vi "DblMonoPMDCurrentScanSM correction 2.vi"() -> ()   [LabVIEW 2009]
uses:
  <vilib>/DAQmx/create/channels.llb/DAQmx Create Channel (AI-Voltage-Basic).vi
  <vilib>/DAQmx/create/channels.llb/DAQmx Create Channel (AO-Voltage-Basic).vi
  <vilib>/DAQmx/write.llb/DAQmx Write (Analog DBL 1Chan 1Samp).vi
  <vilib>/DAQmx/read.llb/DAQmx Read (Analog 1D DBL 1Chan NSamp).vi
  <vilib>/DAQmx/configure/timing.llb/DAQmx Timing (Sample Clock).vi
  <vilib>/DAQmx/read.llb/DAQmx Read (Analog 1D DBL NChan 1Samp).vi
  <vilib>/DAQmx/write.llb/DAQmx Write (Analog 1D DBL 1Chan NSamp).vi
  <vilib>/Utility/file.llb/Write To Spreadsheet File (DBL).vi
  <vilib>/Analysis/NI_AALBase.lvlib
panel:
  in  "Scan mirrors out 2":tag
  out "initial y 2":dbl
  out "Final Y 2":dbl
  out "Final Y":dbl
  out "initial y":dbl
  in  "Volts/pixel":dbl
  out "Xin":dbl
  out "Yin":dbl
  in  "Correction":dbl[][](array[numeric])
  in  "Scan mirrors out":tag
  in  "Scan Mirrors in":tag
  in  "Voltage B":dbl min=-10.0 max=10.0 step=0.1 format="%0.2f"
  in  "Voltage A":dbl min=-10.0 max=10.0 step=0.1 format="%0.2f"
  in  "Output B":tag="Dev1/ao3"
  in  "Output A":tag="Dev1/ao2"
  in  "Input Channel":tag="Dev1/ai6"
  in  "Current":bool
  in  "Power":bool=TRUE
  out "ScanGraph":cluster{dbl[], dbl[]}(graph)
  in  "Sensitivity":dbl=1e-09 caption="(A/V)" format="%#_6p"
  out "Readout":dbl=-2.45576047e-07 format="%^#_9e"
  in  "Scan Save Path":path
  in  "On":bool=TRUE
  out "Waveform Chart":dbl(graph)=-2.45576047e-07
  in  "Save":bool=TRUE
  in  "Exit":bool
  in  "STOP":bool
  in  "Step Time (sec)":dbl=1.0 min=0.001 max=300.0 step=0.001 format="%.3f"
  in  "Step Size (nm)":dbl=1.0 min=0.1 max=100.0 step=0.1 format="%.1f"
  in  "End":dbl=800.0 min=0.0 max=2000.0 step=0.1 format="%.1f"
  in  "Start":dbl=400.0 min=0.0 max=2000.0 step=0.1 format="%.1f"
  in  "Scan":bool
  in  "Up":bool=TRUE caption="Down"
  in  "Increment (nm)":dbl=10.0 min=0.1 max=2000.0 step=0.1 format="%.1f"
  in  "PMD Settings":T1={"Beam Diameter (mm)"=4.0, "BWIn"=0, "Averaging Rate"=300, "Auto Range"=TRUE} {"Averaging Rate" min=33 max=5000 step=1; "BWIn" items=["HIGH", "LOW"]; "Beam Diameter (mm)" min=1.0 max=9.0 step=0.5}
  in  "Step":bool
  out "Busy":bool=TRUE
  in  "Send Command":bool
  in  "Command":u16(ring)=1 items=["nm", "goto", "nm/min", "VIS grating", "IR grating"]
  in  "Wavelength (nm)":dbl=500.0 min=0.0 max=2000.0 step=0.1 format="%.1f"
  in  "Scan Speed (nm/min)":dbl=100.0 min=1.0 max=500.0 step=0.1 format="%.1f"
  out "Done?":string="   ..."
  in  "Send Question":bool
  in  "Ask?":u16(ring) items=["?nm", "?nm/min", "?grating", "?turret", "?gratings"]
  in  "Zero?":bool
  out "PM Error log":string="-222,\"Data out of range\"\n-222,\"Data out of range\"\n-222,\"Data out of range\"\n-222,\"Data out of range\"\n-222,\"Data out of range\"\n-222,\"Data out of range\"\n-222,\"Data out of range\"\n-222,\"Data out of range\"\n-222,\"Data out of range\"\n-222,\"Data out of range\"\n-222,\"Data out of range\"\n-222,\"Data out of range\"\n-222,\"Data out of range\"\n-222,\"Data out of range\"\n-222,\"Data out of range\"\n-222,\"Data out of range\"\n-222,\"Data out of range\"\n-222,\"Data out of range\"\n-222,\"Data out of range\"\n-222,\"Data out of range\"\n-222,\"Data out of range\"\n-222,\"Data out of range\"\n-222,\"Data out of range\"\n-222,\"Data out of range\"\n-222,\"Data out of range\"\n-222,\"Data out of range\"\n-222,\"Data out of range\"\n-222,\"Data out of range\"\n-222,\"Data out of range\"\n-222,\"Data out of range\"\n-222,\"Data out of range\"\n-222,\"Data out of range\"\n-222,\"Data out of range\"\n-222,\"Data out of range\"\n-222,\"Data out of range\"\n-222,\"Data out of range\"\n-222,\"Data out of range\"\n-222,\"Data out of range\"\n-222,\"Data out of range\"\n-222,\"Data out of range\"\n-222,\"Data out of range\"\n-222,\"Data out of range\"\n-222,\"Data out of range\"\n-222,\"Data out of range\"\n-222,\"Data out of range\"\n-222,\"Data out of range\"\n-222,\"Data out of range\"\n-222,\"Data out of range\"\n-222,\"Data out of range\"\n-222,\"Data out of range\"\n-222,\"Data out of range\"\n-222,\"Data out of range\"\n-222,\"Data out of range\"\n-222,\"Data out of range\"\n-222,\"Data out of range\"\n-222,\"Data out of range\"\n-222,\"Data out of range\"\n-222,\"Data out of range\"\n-222,\"Data out of range\"\n-222,\"Data out of range\"\n-222,\"Data out of range\"\n-222,\"Data out of range\"\n-222,\"Data out of range\"\n-222,\"Data out of range\"\n-222,\"Data out of range\"\n-222,\"Data out of range\"\n-222,\"Data out of range\"\n-222,\"Data out of range\"\n-222,\"Data out of range\"\n-222,\"Data out of range\"\n-222,\"Data out of range\"\n-222,\"Data out of range\"\n-222,\"Data out of range\"\n-222,\"Data out of range\"\n-222,\"Data out of range\"\n-222,\"Data out of range\"\n-222,\"Data out of range\"\n-222,\"Data out of range\"\n-222,\"Data out of range\"\n-222,\"Data out of range\"\n-222,\"Data out of range\"\n-222,\"Data out of range\"\n-222,\"Data out of range\"\n-222,\"Data out of range\"\n-222,\"Data out of range\"\n-222,\"Data out of range\"\n-222,\"Data out of range\"\n-222,\"Data out of range\"\n-222,\"Data out of range\"\n-222,\"Data out of range\"\n-222,\"Data out of range\"\n-222,\"Data out of range\"\n-222,\"Data out of range\"\n-222,\"Data out of range\"\n-222,\"Data out of range\"\n-222,\"Data out of range\"\n-222,\"Data out of range\"\n-222,\"Data out of range\"\n-222,\"Data out of range\"\n-222,\"Data out of range\"\n-222,\"Data out of range\"\n-222,\"Data out of range\"\n-222,\"Data out of range\"\n-222,\"Data out of range\"\n-222,\"Data out of range\"\n-222,\"Data out of range\"\n-222,\"Data out of range\"\n-222,\"Data out of range\"\n-222,\"Data out of range\"\n-222,\"Data out of range\"\n-222,\"Data out of range\"\n-222,\"Data out of range\"\n-222,\"Data out of range\"\n-222,\"Data out of range\"\n-222,\"Data out of range\"\n-222,\"Data out of range\"\n-222,\"Data out of range\"\n-222,\"Data out of range\"\n-222,\"Data out of range\"\n-222,\"Data out of range\"\n-222,\"Data out of range\"\n-222,\"Data out of range\"\n-222,\"Data out of range\"\n-222,\"Data out of range\"\n-222,\"Data out of range\"\n-222,\"Data out of range\"\n-222,\"Data out of range\"\n-222,\"Data out of range\"\n-222,\"Data out of range\"\n-222,\"Data out of range\"\n-222,\"Data out of range\"\n-222,\"Data out of range\"\n-222,\"Data out of range\"\n-222,\"Data out of range\"\n-222,\"Data out of range\"\n-222,\"Data out of range\"\n-222,\"Data out of range\"\n-222,\"Data out of range\"\n-222,\"Data out of range\"\n-222,\"Data out of range\"\n-222,\"Data out of range\"\n-222,\"Data out of range\"\n-222,\"Data out of range\"\n-222,\"Data out of range\"\n-222,\"Data out of range\"\n-222,\"Data out of range\"\n-222,\"Data out of range\"\n-222,\"Data out of range\"\n-222,\"Data out of range\"\n-222,\"Data out of range\"\n-222,\"Data out of range\"\n-222,\"Data out of range\"\n-222,\"Data out of range\"\n-222,\"Data out of range\"\n-222,\"Data out of range\"\n-222,\"Data out of range\"\n-222,\"Data out of range\"\n-222,\"Data out of range\"\n-222,\"Data out of range\"\n-222,\"Data out of range\"\n-222,\"Data out of range\"\n-222,\"Data out of range\"\n-222,\"Data out of range\"\n-222,\"Data out of range\"\n-222,\"Data out of range\"\n-222,\"Data out of range\"\n-222,\"Data out of range\"\n-222,\"Data out of range\"\n-222,\"Data out of range\"\n-222,\"Data out of range\"\n-222,\"Data out of range\"\n-222,\"Data out of range\"\n-222,\"Data out of range\"\n-222,\"Data out of range\"\n-222,\"Data out of range\"\n-222,\"Data out of range\"\n-222,\"Data out of range\"\n-222,\"Data out of range\"\n-222,\"Data out of range\"\n-222,\"Data out of range\"\n-222,\"Data out of range\"\n-222,\"Data out of range\"\n-222,\"Data out of range\"\n-222,\"Data out of range\"\n-222,\"Data out of range\"\n-222,\"Data out of range\"\n-222,\"Data out of range\"\n-222,\"Data out of range\"\n-222,\"Data out of range\"\n-222,\"Data out of range\"\n-222,\"Data out of range\"\n-222,\"Data out of range\"\n-222,\"Data out of range\"\n-222,\"Data out of range\"\n-222,\"Data out of range\"\n-222,\"Data out of range\"\n-222,\"Data out of range\"\n-222,\"Data out of range\"\n-222,\"Data out of range\"\n-222,\"Data out of range\"\n-222,\"Data out of range\"\n-222,\"Data out of range\"\n-222,\"Data out of range\"\n-222,\"Data out of range\"\n-222,\"Data out of range\"\n-222,\"Data out of range\"\n-222,\"Data out of range\"\n-222,\"Data out of range\"\n-222,\"Data out of range\"\n-222,\"Data out of range\"\n-222,\"Data out of range\"\n-222,\"Data out of range\"\n-222,\"Data out of range\"\n-222,\"Data out of range\"\n-222,\"Data out of range\"\n-222,\"Data out of range\"\n-222,\"Data out of range\"\n-222,\"Data out of range\"\n-222,\"Data out of range\"\n-222,\"Data out of range\"\n-222,\"Data out of range\"\n-222,\"Data out of range\"\n-222,\"Data out of range\"\n-222,\"Data out of range\"\n-222,\"Data out of range\"\n-222,\"Data out of range\"\n-222,\"Data out of range\"\n-222,\"Data out of range\"\n-222,\"Data out of range\"\n-222,\"Data out of range\"\n-222,\"Data out of range\"\n-222,\"Data out of range\"\n-222,\"Data out of range\"\n-222,\"Data out of range\"\n-222,\"Data out of range\"\n-222,\"Data out of range\"\n-222,\"Data out of range\"\n-222,\"Data out of range\"\n-222,\"Data out of range\"\n-222,\"Data out of range\"\n-222,\"Data out of range\"\n-222,\"Data out of range\"\n-222,\"Data out of range\"\n-222,\"Data out of range\"\n-222,\"Data out of range\"\n-222,\"Data out of range\"\n-222,\"Data out of range\"\n-222,\"Data out of range\"\n-222,\"Data out of range\"\n-222,\"Data out of range\"\n-222,\"Data out of range\"\n-222,\"Data out of range\"\n-222,\"Data out of range\"\n-222,\"Data out of range\"\n-222,\"Data out of range\"\n-222,\"Data out of range\"\n-222,\"Data out of range\"\n-222,\"Data out of range\"\n-222,\"Data out of range\"\n-222,\"Data out of range\"\n-222,\"Data out of range\"\n-222,\"Data out of range\"\n-222,\"Data out of range\"\n-222,\"Data out of range\"\n-222,\"Data out of range\"\n-222,\"Data out of range\"\n-222,\"Data out of range\"\n-222,\"Data out of range\"\n-222,\"Data out of range\"\n-222,\"Data out of range\"\n-222,\"Data out of range\"\n-222,\"Data out of range\"\n-222,\"Data out of range\"\n-222,\"Data out of range\"\n-222,\"Data out of range\"\n-222,\"Data out of range\"\n-222,\"Data out of range\"\n-222,\"Data out of range\"\n-222,\"Data out of range\"\n-222,\"Data out of range\"\n-222,\"Data out of range\"\n-222,\"Data out of range\"\n-222,\"Data out of range\"\n-222,\"Data out of range\"\n-222,\"Data out of range\"\n-222,\"Data out of range\"\n-222,\"Data out of range\"\n-222,\"Data out of range\"\n-222,\"Data out of range\"\n-222,\"Data out of range\"\n-222,\"Data out of range\"\n-222,\"Data out of range\"\n-222,\"Data out of range\"\n-222,\"Data out of range\"\n-222,\"Data out of range\"\n-222,\"Data out of range\"\n-222,\"Data out of range\"\n-222,\"Data out of range\"\n-222,\"Data out of range\"\n-222,\"Data out of range\"\n-222,\"Data out of range\"\n-222,\"Data out of range\"\n-222,\"Data out of range\"\n-222,\"Data out of range\"\n-222,\"Data out of range\"\n-222,\"Data out of range\"\n-222,\"Data out of range\"\n-222,\"Data out of range\"\n-222,\"Data out of range\"\n-222,\"Data out of range\"\n-222,\"Data out of range\"\n-222,\"Data out of range\"\n-222,\"Data out of range\"\n-222,\"Data out of range\"\n-222,\"Data out of range\"\n-222,\"Data out of range\"\n-222,\"Data out of range\"\n-222,\"Data out of range\"\n-222,\"Data out of range\"\n-222,\"Data out of range\"\n-222,\"Data out of range\"\n-222,\"Data out of range\"\n-222,\"Data out of range\"\n-222,\"Data out of range\"\n-222,\"Data out of range\"\n-222,\"Data out of range\"\n-222,\"Data out of range\"\n-222,\"Data out of range\"\n-222,\"Data out of range\"\n-222,\"Data out of range\"\n-222,\"Data out of range\"\n-222,\"Data out of range\"\n-222,\"Data out of range\"\n-222,\"Data out of range\"\n-222,\"Data out of range\"\n-222,\"Data out of range\"\n-222,\"Data out of range\"\n-222,\"Data out of range\"\n-222,\"Data out of range\"\n-222,\"Data out of range\"\n-222,\"Data out of range\"\n-222,\"Data out of range\"\n-222,\"Data out of range\"\n-222,\"Data out of range\"\n-222,\"Data out of range\"\n-222,\"Data out of range\"\n-222,\"Data out of range\"\n-222,\"Data out of range\"\n-222,\"Data out of range\"\n-222,\"Data out of range\"\n-222,\"Data out of range\"\n-222,\"Data out of range\"\n-222,\"Data out of range\"\n-222,\"Data out of range\"\n-222,\"Data out of range\"\n-222,\"Data out of range\"\n-222,\"Data out of range\"\n-222,\"Data out of range\"\n-222,\"Data out of range\"\n-222,\"Data out of range\"\n-222,\"Data out of range\"\n-222,\"Data out of range\"\n-222,\"Data out of range\"\n-222,\"Data out of range\"\n-222,\"Data out of range\"\n-222,\"Data out of range\"\n-222,\"Data out of range\"\n-222,\"Data out of range\"\n-222,\"Data out of range\"\n-222,\"Data out of range\"\n-222,\"Data out of range\"\n-222,\"Data out of range\"\n-222,\"Data out of range\"\n-222,\"Data out of range\"\n-222,\"Data out of range\"\n-222,\"Data out of range\"\n-222,\"Data out of range\"\n-222,\"Data out of range\"\n-222,\"Data out of range\"\n-222,\"Data out of range\"\n-222,\"Data out of range\"\n-222,\"Data out of range\"\n-222,\"Data out of range\"\n-222,\"Data out of range\"\n-222,\"Data out of range\"\n-222,\"Data out of range\"\n-222,\"Data out of range\"\n-222,\"Data out of range\"\n-222,\"Data out of range\"\n-222,\"Data out of range\"\n-222,\"Data out of range\"\n-222,\"Data out of range\"\n-222,\"Data out of range\"\n-222,\"Data out of range\"\n-222,\"Data out of range\"\n-222,\"Data out of range\"\n-222,\"Data out of range\"\n-222,\"Data out of range\"\n-222,\"Data out of range\"\n-222,\"Data out of range\"\n-222,\"Data out of range\"\n-222,\"Data out of range\"\n-222,\"Data out of range\"\n-222,\"Data out of range\"\n-222,\"Data out of range\"\n-222,\"Data out of range\"\n-222,\"Data out of range\"\n-222,\"Data out of range\"\n-222,\"Data out of range\"\n-222,\"Data out of range\"\n-222,\"Data out of range\"\n-222,\"Data out of range\"\n-222,\"Data out of range\"\n-222,\"Data out of range\"\n-222,\"Data out of range\"\n-222,\"Data out of range\"\n-222,\"Data out of range\"\n-222,\"Data out of range\"\n-222,\"Data out of range\"\n-222,\"Data out of range\"\n-222,\"Data out of range\"\n-222,\"Data out of range\"\n-222,\"Data out of range\"\n-222,\"Data out of range\"\n-222,\"Data out of range\"\n-222,\"Data out of range\"\n-222,\"Data out of range\"\n-222,\"Data out of range\"\n-222,\"Data out of range\"\n-222,\"Data out of range\"\n-222,\"Data out of range\"\n-222,\"Data out of range\"\n-222,\"Data out of range\"\n-222,\"Data out of range\"\n-222,\"Data out of range\"\n-222,\"Data out of range\"\n-222,\"Data out of range\"\n-222,\"Data out of range\"\n-222,\"Data out of range\"\n-222,\"Data out of range\"\n-222,\"Data out of range\"\n-222,\"Data out of range\"\n-222,\"Data out of range\"\n-222,\"Data out of range\"\n-222,\"Data out of range\"\n-222,\"Data out of range\"\n-222,\"Data out of range\"\n-222,\"Data out of range\"\n-222,\"Data out of range\"\n-222,\"Data out of range\"\n-222,\"Data out of range\"\n-222,\"Data out of range\"\n-222,\"Data out of range\"\n-222,\"Data out of range\"\n-222,\"Data out of range\"\n-222,\"Data out of range\"\n-222,\"Data out of range\"\n-222,\"Data out of range\"\n-222,\"Data out of range\"\n-222,\"Data out of range\"\n-222,\"Data out of range\"\n-222,\"Data out of range\"\n-222,\"Data out of range\"\n-222,\"Data out of range\"\n-222,\"Data out of range\"\n-222,\"Data out of range\"\n-222,\"Data out of range\"\n-222,\"Data out of range\"\n-222,\"Data out of range\"\n-222,\"Data out of range\"\n-222,\"Data out of range\"\n-222,\"Data out of range\"\n-222,\"Data out of range\"\n-222,\"Data out of range\"\n-222,\"Data out of range\"\n-222,\"Data out of range\"\n-222,\"Data out of range\"\n-222,\"Data out of range\"\n-222,\"Data out of range\"\n-222,\"Data out of range\"\n-222,\"Data out of range\"\n-222,\"Data out of range\"\n-222,\"Data out of range\"\n-222,\"Data out of range\"\n-222,\"Data out of range\"\n-222,\"Data out of range\"\n-222,\"Data out of range\"\n-222,\"Data out of range\"\n-222,\"Data out of range\"\n-222,\"Data out of range\"\n-222,\"Data out of range\"\n-222,\"Data out of range\"\n-222,\"Data out of range\"\n-222,\"Data out of range\"\n-222,\"Data out of range\"\n-222,\"Data out of range\"\n-222,\"Data out of range\"\n-222,\"Data out of range\"\n-222,\"Data out of range\"\n-222,\"Data out of range\"\n-222,\"Data out of range\"\n-222,\"Data out of range\"\n-222,\"Data out of range\"\n-222,\"Data out of range\"\n-222,\"Data out of range\"\n-222,\"Data out of range\"\n-222,\"Data out of range\"\n-222,\"Data out of range\"\n-222,\"Data out of range\"\n-222,\"Data out of range\"\n-222,\"Data out of range\"\n-222,\"Data out of range\"\n-222,\"Data out of range\"\n-222,\"Data out of range\"\n-222,\"Data out of range\"\n-222,\"Data out of range\"\n-222,\"Data out of range\"\n-222,\"Data out of range\"\n-222,\"Data out of range\"\n-222,\"Data out of range\"\n-222,\"Data out of range\"\n-222,\"Data out of range\"\n-222,\"Data out of range\"\n-222,\"Data out of range\"\n-222,\"Data out of range\"\n-222,\"Data out of range\"\n-222,\"Data out of range\"\n-222,\"Data out of range\"\n-222,\"Data out of range\"\n-222,\"Data out of range\"\n-222,\"Data out of range\"\n-222,\"Data out of range\"\n-222,\"Data out of range\"\n-222,\"Data out of range\"\n-222,\"Data out of range\"\n-222,\"Data out of range\"\n-222,\"Data out of range\"\n-222,\"Data out of range\"\n-222,\"Data out of range\"\n-222,\"Data out of range\"\n-222,\"Data out of range\"\n-222,\"Data out of range\"\n-222,\"Data out of range\"\n-222,\"Data out of range\"\n-222,\"Data out of range\"\n-222,\"Data out of range\"\n-222,\"Data out of range\"\n-222,\"Data out of range\"\n-222,\"Data out of range\"\n-222,\"Data out of range\"\n-222,\"Data out of range\"\n-222,\"Data out of range\"\n-222,\"Data out of range\"\n-222,\"Data out of range\"\n-222,\"Data out of range\"\n-222,\"Data out of range\"\n-222,\"Data out of range\"\n-222,\"Data out of range\"\n-222,\"Data out of range\"\n-222,\"Data out of range\"\n-222,\"Data out of range\"\n-222,\"Data out of range\"\n-222,\"Data out of range\"\n-222,\"Data out of range\"\n-222,\"Data out of range\"\n-222,\"Data out of range\"\n-222,\"Data out of range\"\n-222,\"Data out of range\"\n-222,\"Data out of range\"\n-222,\"Data out of range\"\n-222,\"Data out of range\"\n-222,\"Data out of range\"\n-222,\"Data out of range\"\n-222,\"Data out of range\"\n-222,\"Data out of range\"\n-222,\"Data out of range\"\n-222,\"Data out of range\"\n-222,\"Data out of range\"\n-222,\"Data out of range\"\n-222,\"Data out of range\"\n-222,\"Data out of range\"\n-222,\"Data out of range\"\n-222,\"Data out of range\"\n-222,\"Data out of range\"\n-222,\"Data out of range\"\n-222,\"Data out of range\"\n-222,\"Data out of range\"\n-222,\"Data out of range\"\n-222,\"Data out of range\"\n-222,\"Data out of range\"\n-222,\"Data out of range\"\n-222,\"Data out of range\"\n-222,\"Data out of range\"\n-222,\"Data out of range\"\n-222,\"Data out of range\"\n-222,\"Data out of range\"\n-222,\"Data out of range\"\n-222,\"Data out of range\"\n-222,\"Data out of range\"\n-222,\"Data out of range\"\n-222,\"Data out of range\"\n-222,\"Data out of range\"\n-222,\"Data out of range\"\n-222,\"Data out of range\"\n-222,\"Data out of range\"\n-222,\"Data out of range\"\n-222,\"Data out of range\"\n-222,\"Data out of range\"\n-222,\"Data out of range\"\n-222,\"Data out of range\"\n-222,\"Data out of range\"\n-222,\"Data out of range\"\n-222,\"Data out of range\"\n-222,\"Data out of range\"\n-222,\"Data out of range\"\n-222,\"Data out of range\"\n-222,\"Data out of range\"\n-222,\"Data out of range\"\n-222,\"Data out of range\"\n-222,\"Data out of range\"\n-222,\"Data out of range\"\n-222,\"Data out of range\"\n-222,\"Data out of range\"\n-222,\"Data out of range\"\n-222,\"Data out of range\"\n-222,\"Data out of range\"\n-222,\"Data out of range\"\n-222,\"Data out of range\"\n-222,\"Data out of range\"\n-222,\"Data out of range\"\n-222,\"Data out of range\"\n-222,\"Data out of range\"\n-222,\"Data out of range\"\n-222,\"Data out of range\"\n-222,\"Data out of range\"\n-222,\"Data out of range\"\n-222,\"Data out of range\"\n-222,\"Data out of range\"\n-222,\"Data out of range\"\n-222,\"Data out of range\"\n-222,\"Data out of range\"\n-222,\"Data out of range\"\n-222,\"Data out of range\"\n-222,\"Data out of range\"\n-222,\"Data out of range\"\n-222,\"Data out of range\"\n-222,\"Data out of range\"\n-222,\"Data out of range\"\n-222,\"Data out of range\"\n-222,\"Data out of range\"\n-222,\"Data out of range\"\n-222,\"Data out of range\"\n-222,\"Data out of range\"\n-222,\"Data out of range\"\n-222,\"Data out of range\"\n-222,\"Data out of range\"\n-222,\"Data out of range\"\n-222,\"Data out of range\"\n-222,\"Data out of range\"\n-222,\"Data out of range\"\n-222,\"Data out of range\"\n-222,\"Data out of range\"\n-222,\"Data out of range\"\n-222,\"Data out of range\"\n-222,\"Data out of range\"\n-222,\"Data out of range\"\n-222,\"Data out of range\"\n-222,\"Data out of range\"\n-222,\"Data out of range\"\n-222,\"Data out of range\"\n-222,\"Data out of range\"\n-222,\"Data out of range\"\n-222,\"Data out of range\"\n-222,\"Data out of range\"\n-222,\"Data out of range\"\n-222,\"Data out of range\"\n-222,\"Data out of range\"\n-222,\"Data out of range\"\n-222,\"Data out of range\"\n-222,\"Data out of range\"\n-222,\"Data out of range\"\n-222,\"Data out of range\"\n-222,\"Data out of range\"\n-222,\"Data out of range\"\n-222,\"Data out of range\"\n-222,\"Data out of range\"\n-222,\"Data out of range\"\n-222,\"Data out of range\"\n-222,\"Data out of range\"\n-222,\"Data out of range\"\n-222,\"Data out of range\"\n-222,\"Data out of range\"\n-222,\"Data out of range\"\n-222,\"Data out of range\"\n-222,\"Data out of range\"\n-222,\"Data out of range\"\n-222,\"Data out of range\"\n-222,\"Data out of range\"\n-222,\"Data out of range\"\n-222,\"Data out of range\"\n-222,\"Data out of range\"\n-222,\"Data out of range\"\n-222,\"Data out of range\"\n-222,\"Data out of range\"\n-222,\"Data out of range\"\n-222,\"Data out of range\"\n-222,\"Data out of range\"\n-222,\"Data out of range\"\n-222,\"Data out of range\"\n-222,\"Data out of range\"\n-222,\"Data out of range\"\n-222,\"Data out of range\"\n-222,\"Data out of range\"\n-222,\"Data out of range\"\n-222,\"Data out of range\"\n-222,\"Data out of range\"\n-222,\"Data out of range\"\n-222,\"Data out of range\"\n-222,\"Data out of range\"\n-222,\"Data out of range\"\n-222,\"Data out of range\"\n-222,\"Data out of range\"\n-222,\"Data out of range\"\n-222,\"Data out of range\"\n-222,\"Data out of range\"\n-222,\"Data out of range\"\n-222,\"Data out of range\"\n-222,\"Data out of range\"\n-222,\"Data out of range\"\n-222,\"Data out of range\"\n-222,\"Data out of range\"\n-222,\"Data out of range\"\n-222,\"Data out of range\"\n-222,\"Data out of range\"\n-222,\"Data out of range\"\n-222,\"Data out of range\"\n-222,\"Data out of range\"\n-222,\"Data out of range\"\n-222,\"Data out of range\"\n-222,\"Data out of range\"\n-222,\"Data out of range\"\n-222,\"Data out of range\"\n-222,\"Data out of range\"\n-222,\"Data out of range\"\n-222,\"Data out of range\"\n-222,\"Data out of range\"\n-222,\"Data out of range\"\n-222,\"Data out of range\"\n-222,\"Data out of range\"\n-222,\"Data out of range\"\n-222,\"Data out of range\"\n-222,\"Data out of range\"\n-222,\"Data out of range\"\n-222,\"Data out of range\"\n-222,\"Data out of range\"\n-222,\"Data out of range\"\n-222,\"Data out of range\"\n-222,\"Data out of range\"\n-222,\"Data out of range\"\n-222,\"Data out of range\"\n-222,\"Data out of range\"\n-222,\"Data out of range\"\n-222,\"Data out of range\"\n-222,\"Data out of range\"\n-222,\"Data out of range\"\n-222,\"Data out of range\"\n-222,\"Data out of range\"\n-222,\"Data out of range\"\n-222,\"Data out of range\"\n-222,\"Data out of range\"\n-222,\"Data out of range\"\n-222,\"Data out of range\"\n-222,\"Data out of range\"\n-222,\"Data out of range\"\n-222,\"Data out of range\"\n-222,\"Data out of range\"\n-222,\"Data out of range\"\n-222,\"Data out of range\"\n-222,\"Data out of range\"\n-222,\"Data out of range\"\n-222,\"Data out of range\"\n-222,\"Data out of range\"\n-222,\"Data out of range\"\n-222,\"Data out of range\"\n-222,\"Data out of range\"\n-222,\"Data out of range\"\n-222,\"Data out of range\"\n-222,\"Data out of range\"\n-222,\"Data out of range\"\n-222,\"Data out of range\"\n-222,\"Data out of range\"\n-222,\"Data out of range\"\n-222,\"Data out of range\"\n-222,\"Data out of range\"\n-222,\"Data out of range\"\n-222,\"Data out of range\"\n-222,\"Data out of range\"\n-222,\"Data out of range\"\n-222,\"Data out of range\"\n-222,\"Data out of range\"\n-222,\"Data out of range\"\n-222,\"Data out of range\"\n-222,\"Data out of range\"\n-222,\"Data out of range\"\n-222,\"Data out of range\"\n-222,\"Data out of range\"\n-222,\"Data out of range\"\n-222,\"Data out of range\"\n-222,\"Data out of range\"\n-222,\"Data out of range\"\n-222,\"Data out of range\"\n-222,\"Data out of range\"\n-222,\"Data out of range\"\n-222,\"Data out of range\"\n-222,\"Data out of range\"\n-222,\"Data out of range\"\n-222,\"Data out of range\"\n-222,\"Data out of range\"\n-222,\"Data out of range\"\n-222,\"Data out of range\"\n-222,\"Data out of range\"\n-222,\"Data out of range\"\n-222,\"Data out of range\"\n-222,\"Data out of range\"\n-222,\"Data out of range\"\n-222,\"Data out of range\"\n-222,\"Data out of range\"\n-222,\"Data out of range\"\n-222,\"Data out of range\"\n-222,\"Data out of range\"\n-222,\"Data out of range\"\n-222,\"Data out of range\"\n-222,\"Data out of range\"\n-222,\"Data out of range\"\n-222,\"Data out of range\"\n-222,\"Data out of range\"\n-222,\"Data out of range\"\n-222,\"Data out of range\"\n-222,\"Data out of range\"\n-222,\"Data out of range\"\n-222,\"Data out of range\"\n-222,\"Data out of range\"\n-222,\"Data out of range\"\n-222,\"Data out of range\"\n-222,\"Data out of range\"\n-222,\"Data out of range\"\n-222,\"Data out of range\"\n-222,\"Data out of range\"\n-222,\"Data out of range\"\n-222,\"Data out of range\"\n-222,\"Data out of range\"\n-222,\"Data out of range\"\n-222,\"Data out of range\"\n-222,\"Data out of range\"\n-222,\"Data out of range\"\n-222,\"Data out of range\"\n-222,\"Data out of range\"\n-222,\"Data out of range\"\n-222,\"Data out of range\"\n-222,\"Data out of range\"\n-222,\"Data out of range\"\n-222,\"Data out of range\"\n-222,\"Data out of range\"\n-222,\"Data out of range\"\n-222,\"Data out of range\"\n-222,\"Data out of range\"\n-222,\"Data out of range\"\n-222,\"Data out of range\"\n-222,\"Data out of range\"\n-222,\"Data out of range\"\n-222,\"Data out of range\"\n-222,\"Data out of range\"\n-222,\"Data out of range\"\n-222,\"Data out of range\"\n-222,\"Data out of range\"\n-222,\"Data out of range\"\n-222,\"Data out of range\"\n-222,\"Data out of range\"\n-222,\"Data out of range\"\n-222,\"Data out of range\"\n-222,\"Data out of range\"\n-222,\"Data out of range\"\n-222,\"Data out of range\"\n-222,\"Data out of range\"\n-222,\"Data out of range\"\n-222,\"Data out of range\"\n-222,\"Data out of range\"\n-222,\"Data out of range\"\n-222,\"Data out of range\"\n-222,\"Data out of range\"\n-222,\"Data out of range\"\n-222,\"Data out of range\"\n-222,\"Data out of range\"\n-222,\"Data out of range\"\n-222,\"Data out of range\"\n-222,\"Data out of range\"\n-222,\"Data out of range\"\n-222,\"Data out of range\"\n-222,\"Data out of range\"\n-222,\"Data out of range\"\n-222,\"Data out of range\"\n-222,\"Data out of range\"\n-222,\"Data out of range\"\n-222,\"Data out of range\"\n-222,\"Data out of range\"\n-222,\"Data out of range\"\n-222,\"Data out of range\"\n-222,\"Data out of range\"\n-222,\"Data out of range\"\n-222,\"Data out of range\"\n-222,\"Data out of range\"\n-222,\"Data out of range\"\n-222,\"Data out of range\"\n-222,\"Data out of range\"\n-222,\"Data out of range\"\n-222,\"Data out of range\"\n-222,\"Data out of range\"\n-222,\"Data out of range\"\n-222,\"Data out of range\"\n-222,\"Data out of range\"\n-222,\"Data out of range\"\n-222,\"Data out of range\"\n-222,\"Data out of range\"\n-222,\"Data out of range\"\n-222,\"Data out of range\"\n-222,\"Data out of range\"\n-222,\"Data out of range\"\n-222,\"Data out of range\"\n-222,\"Data out of range\"\n-222,\"Data out of range\"\n-222,\"Data out of range\"\n-222,\"Data out of range\"\n-222,\"Data out of range\"\n-222,\"Data out of range\"\n-222,\"Data out of range\"\n-222,\"Data out of range\"\n-222,\"Data out of range\"\n-222,\"Data out of range\"\n-222,\"Data out of range\"\n-222,\"Data out of range\"\n-222,\"Data out of range\"\n-222,\"Data out of range\"\n-222,\"Data out of range\"\n-222,\"Data out of range\"\n-222,\"Data out of range\"\n-222,\"Data out of range\"\n-222,\"Data out of range\"\n-222,\"Data out of range\"\n-222,\"Data out of range\"\n-222,\"Data out of range\"\n-222,\"Data out of range\"\n-222,\"Data out of range\"\n-222,\"Data out of range\"\n-222,\"Data out of range\"\n-222,\"Data out of range\"\n-222,\"Data out of range\"\n-222,\"Data out of range\"\n-222,\"Data out of range\"\n-222,\"Data out of range\"\n-222,\"Data out of range\"\n-222,\"Data out of range\"\n-222,\"Data out of range\"\n-222,\"Data out of range\"\n-222,\"Data out of range\"\n-222,\"Data out of range\"\n-222,\"Data out of range\"\n-222,\"Data out of range\"\n-222,\"Data out of range\"\n-222,\"Data out of range\"\n-222,\"Data out of range\"\n-222,\"Data out of range\"\n-222,\"Data out of range\"\n-222,\"Data out of range\"\n-222,\"Data out of range\"\n-222,\"Data out of range\"\n-222,\"Data out of range\"\n-222,\"Data out of range\"\n-222,\"Data out of range\"\n-222,\"Data out of range\"\n-222,\"Data out of range\"\n-222,\"Data out of range\"\n-222,\"Data out of range\"\n-222,\"Data out of range\"\n-222,\"Data out of range\"\n-222,\"Data out of range\"\n-222,\"Data out of range\"\n-222,\"Data out of range\"\n-222,\"Data out of range\"\n-222,\"Data out of range\"\n-222,\"Data out of range\"\n-222,\"Data out of range\"\n-222,\"Data out of range\"\n-222,\"Data out of range\"\n-222,\"Data out of range\"\n-222,\"Data out of range\"\n-222,\"Data out of range\"\n-222,\"Data out of range\"\n-222,\"Data out of range\"\n-222,\"Data out of range\"\n-222,\"Data out of range\"\n-222,\"Data out of range\"\n-222,\"Data out of range\"\n-222,\"Data out of range\"\n-222,\"Data out of range\"\n-222,\"Data out of range\"\n-222,\"Data out of range\"\n-222,\"Data out of range\"\n-222,\"Data out of range\"\n-222,\"Data out of range\"\n-222,\"Data out of range\"\n-222,\"Data out of range\"\n-222,\"Data out of range\"\n-222,\"Data out of range\"\n-222,\"Data out of range\"\n-222,\"Data out of range\"\n-222,\"Data out of range\"\n-222,\"Data out of range\"\n-222,\"Data out of range\"\n-222,\"Data out of range\"\n-222,\"Data out of range\"\n-222,\"Data out of range\"\n-222,\"Data out of range\"\n-222,\"Data out of range\"\n-222,\"Data out of range\"\n-222,\"Data out of range\"\n-222,\"Data out of range\"\n-222,\"Data out of range\"\n-222,\"Data out of range\"\n-222,\"Data out of range\"\n-222,\"Data out of range\"\n-222,\"Data out of range\"\n-222,\"Data out of range\"\n-222,\"Data out of range\"\n-222,\"Data out of range\"\n-222,\"Data out of range\"\n-222,\"Data out of range\"\n-222,\"Data out of range\"\n-222,\"Data out of range\"\n-222,\"Data out of range\"\n-222,\"Data out of range\"\n-222,\"Data out of range\"\n-222,\"Data out of range\"\n-222,\"Data out of range\"\n-222,\"Data out of range\"\n-222,\"Data out of range\"\n-222,\"Data out of range\"\n-222,\"Data out of range\"\n-222,\"Data out of range\"\n-222,\"Data out of range\"\n-222,\"Data out of range\"\n-222,\"Data out of range\"\n-222,\"Data out of range\"\n-222,\"Data out of range\"\n-222,\"Data out of range\"\n-222,\"Data out of range\"\n-222,\"Data out of range\"\n-222,\"Data out of range\"\n-222,\"Data out of range\"\n-222,\"Data out of range\"\n-222,\"Data out of range\"\n-222,\"Data out of range\"\n-222,\"Data out of range\"\n-222,\"Data out of range\"\n-222,\"Data out of range\"\n-222,\"Data out of range\"\n-222,\"Data out of range\"\n-222,\"Data out of range\"\n-222,\"Data out of range\"\n-222,\"Data out of range\"\n-222,\"Data out of range\"\n-222,\"Data out of range\"\n-222,\"Data out of range\"\n-222,\"Data out of range\"\n-222,\"Data out of range\"\n-222,\"Data out of range\"\n-222,\"Data out of range\"\n-222,\"Data out of range\"\n-222,\"Data out of range\"\n-222,\"Data out of range\"\n-222,\"Data out of range\"\n-222,\"Data out of range\"\n-222,\"Data out of range\"\n-222,\"Data out of range\"\n-222,\"Data out of range\"\n-222,\"Data out of range\"\n-222,\"Data out of range\"\n-222,\"Data out of range\"\n-222,\"Data out of range\"\n-222,\"Data out of range\"\n-222,\"Data out of range\"\n-222,\"Data out of range\"\n-222,\"Data out of range\"\n-222,\"Data out of range\"\n-222,\"Data out of range\"\n-222,\"Data out of range\"\n-222,\"Data out of range\"\n-222,\"Data out of range\"\n-222,\"Data out of range\"\n-222,\"Data out of range\"\n-222,\"Data out of range\"\n-222,\"Data out of range\"\n-222,\"Data out of range\"\n-222,\"Data out of range\"\n-222,\"Data out of range\"\n-222,\"Data out of range\"\n-222,\"Data out of range\"\n-222,\"Data out of range\"\n-222,\"Data out of range\"\n-222,\"Data out of range\"\n-222,\"Data out of range\"\n-222,\"Data out of range\"\n-222,\"Data out of range\"\n-222,\"Data out of range\"\n-222,\"Data out of range\"\n-222,\"Data out of range\"\n-222,\"Data out of range\"\n-222,\"Data out of range\"\n-222,\"Data out of range\"\n-222,\"Data out of range\"\n-222,\"Data out of range\"\n-222,\"Data out of range\"\n-222,\"Data out of range\"\n-222,\"Data out of range\"\n-222,\"Data out of range\"\n-222,\"Data out of range\"\n-222,\"Data out of range\"\n-222,\"Data out of range\"\n-222,\"Data out of range\"\n-222,\"Data out of range\"\n-222,\"Data out of range\"\n-222,\"Data out of range\"\n-222,\"Data out of range\"\n-222,\"Data out of range\"\n-222,\"Data out of range\"\n-222,\"Data out of range\"\n-222,\"Data out of range\"\n-222,\"Data out of range\"\n-222,\"Data out of range\"\n-222,\"Data out of range\"\n-222,\"Data out of range\"\n-222,\"Data out of range\"\n-222,\"Data out of range\"\n-222,\"Data out of range\"\n-222,\"Data out of range\"\n-222,\"Data out of range\"\n-222,\"Data out of range\"\n-222,\"Data out of range\"\n-222,\"Data out of range\"\n-222,\"Data out of range\"\n-222,\"Data out of range\"\n-222,\"Data out of range\"\n-222,\"Data out of range\"\n-222,\"Data out of range\"\n-222,\"Data out of range\"\n-222,\"Data out of range\"\n-222,\"Data out of range\"\n-222,\"Data out of range\"\n-222,\"Data out of range\"\n-222,\"Data out of range\"\n-222,\"Data out of range\"\n-222,\"Data out of range\"\n-222,\"Data out of range\"\n-222,\"Data out of range\"\n-222,\"Data out of range\"\n-222,\"Data out of range\"\n-222,\"Data out of range\"\n-222,\"Data out of range\"\n-222,\"Data out of range\"\n-222,\"Data out of range\"\n-222,\"Data out of range\"\n-222,\"Data out of range\"\n-222,\"Data out of range\"\n-222,\"Data out of range\"\n-222,\"Data out of range\"\n-222,\"Data out of range\"\n-222,\"Data out of range\"\n-222,\"Data out of range\"\n-222,\"Data out of range\"\n-222,\"Data out of range\"\n-222,\"Data out of range\"\n-222,\"Data out of range\"\n-222,\"Data out of range\"\n-222,\"Data out of range\"\n-222,\"Data out of range\"\n-222,\"Data out of range\"\n-222,\"Data out of range\"\n-222,\"Data out of range\"\n-222,\"Data out of range\"\n-222,\"Data out of range\"\n-222,\"Data out of range\"\n-222,\"Data out of range\"\n-222,\"Data out of range\"\n-222,\"Data out of range\"\n-222,\"Data out of range\"\n-222,\"Data out of range\"\n-222,\"Data out of range\"\n-222,\"Data out of range\"\n-222,\"Data out of range\"\n-222,\"Data out of range\"\n-222,\"Data out of range\"\n-222,\"Data out of range\"\n-222,\"Data out of range\"\n-222,\"Data out of range\"\n-222,\"Data out of range\"\n-222,\"Data out of range\"\n-222,\"Data out of range\"\n-222,\"Data out of range\"\n-222,\"Data out of range\"\n-222,\"Data out of range\"\n-222,\"Data out of range\"\n-222,\"Data out of range\"\n-222,\"Data out of range\"\n-222,\"Data out of range\"\n-222,\"Data out of range\"\n-222,\"Data out of range\"\n-222,\"Data out of range\"\n-222,\"Data out of range\"\n-222,\"Data out of range\"\n-222,\"Data out of range\"\n-222,\"Data out of range\"\n-222,\"Data out of range\"\n-222,\"Data out of range\"\n-222,\"Data out of range\"\n-222,\"Data out of range\"\n-222,\"Data out of range\"\n-222,\"Data out of range\"\n-222,\"Data out of range\"\n-222,\"Data out of range\"\n-222,\"Data out of range\"\n-222,\"Data out of range\"\n-222,\"Data out of range\"\n-222,\"Data out of range\"\n-222,\"Data out of range\"\n-222,\"Data out of range\"\n-222,\"Data out of range\"\n-222,\"Data out of range\"\n-222,\"Data out of range\"\n-222,\"Data out of range\"\n-222,\"Data out of range\"\n-222,\"Data out of range\"\n-222,\"Data out of range\"\n-222,\"Data out of range\"\n-222,\"Data out of range\"\n-222,\"Data out of range\"\n-222,\"Data out of range\"\n-222,\"Data out of range\"\n-222,\"Data out of range\"\n-222,\"Data out of range\"\n-222,\"Data out of range\"\n-222,\"Data out of range\"\n-222,\"Data out of range\"\n-222,\"Data out of range\"\n-222,\"Data out of range\"\n-222,\"Data out of range\"\n-222,\"Data out of range\"\n-222,\"Data out of range\"\n-222,\"Data out of range\"\n-222,\"Data out of range\"\n-222,\"Data out of range\"\n-222,\"Data out of range\"\n-222,\"Data out of range\"\n-222,\"Data out of range\"\n-222,\"Data out of range\"\n-222,\"Data out of range\"\n-222,\"Data out of range\"\n-222,\"Data out of range\"\n-222,\"Data out of range\"\n-222,\"Data out of range\"\n-222,\"Data out of range\"\n-222,\"Data out of range\"\n-222,\"Data out of range\"\n-222,\"Data out of range\"\n-222,\"Data out of range\"\n-222,\"Data out of range\"\n-222,\"Data out of range\"\n-222,\"Data out of range\"\n-222,\"Data out of range\"\n-222,\"Data out of range\"\n-222,\"Data out of range\"\n-222,\"Data out of range\"\n-222,\"Data out of range\"\n-222,\"Data out of range\"\n-222,\"Data out of range\"\n-222,\"Data out of range\"\n-222,\"Data out of range\"\n-222,\"Data out of range\"\n-222,\"Data out of range\"\n-222,\"Data out of range\"\n-222,\"Data out of range\"\n-222,\"Data out of range\"\n-222,\"Data out of range\"\n-222,\"Data out of range\"\n-222,\"Data out of range\"\n-222,\"Data out of range\"\n-222,\"Data out of range\"\n-222,\"Data out of range\"\n-222,\"Data out of range\"\n-222,\"Data out of range\"\n-222,\"Data out of range\"\n-222,\"Data out of range\"\n-222,\"Data out of range\"\n-222,\"Data out of range\"\n-222,\"Data out of range\"\n-222,\"Data out of range\"\n-222,\"Data out of range\"\n-222,\"Data out of range\"\n-222,\"Data out of range\"\n-222,\"Data out of range\"\n-222,\"Data out of range\"\n-222,\"Data out of range\"\n-222,\"Data out of range\"\n-222,\"Data out of range\"\n-222,\"Data out of range\"\n-222,\"Data out of range\"\n-222,\"Data out of range\"\n-222,\"Data out of range\"\n-222,\"Data out of range\"\n-222,\"Data out of range\"\n-222,\"Data out of range\"\n-222,\"Data out of range\"\n-222,\"Data out of range\"\n-222,\"Data out of range\"\n-222,\"Data out of range\"\n-222,\"Data out of range\"\n-222,\"Data out of range\"\n-222,\"Data out of range\"\n-222,\"Data out of range\"\n-222,\"Data out of range\"\n-222,\"Data out of range\"\n-222,\"Data out of range\"\n-222,\"Data out of range\"\n-222,\"Data out of range\"\n-222,\"Data out of range\"\n-222,\"Data out of range\"\n-222,\"Data out of range\"\n-222,\"Data out of range\"\n-222,\"Data out of range\"\n-222,\"Data out of range\"\n-222,\"Data out of range\"\n-222,\"Data out of range\"\n-222,\"Data out of range\"\n-222,\"Data out of range\"\n-222,\"Data out of range\"\n-222,\"Data out of range\"\n-222,\"Data out of range\"\n-222,\"Data out of range\"\n-222,\"Data out of range\"\n-222,\"Data out of range\"\n-222,\"Data out of range\"\n-222,\"Data out of range\"\n-222,\"Data out of range\"\n-222,\"Data out of range\"\n-222,\"Data out of range\"\n-222,\"Data out of range\"\n-222,\"Data out of range\"\n-222,\"Data out of range\"\n-222,\"Data out of range\"\n-222,\"Data out of range\"\n-222,\"Data out of range\"\n-222,\"Data out of range\"\n-222,\"Data out of range\"\n-222,\"Data out of range\"\n-222,\"Data out of range\"\n-222,\"Data out of range\"\n-222,\"Data out of range\"\n-222,\"Data out of range\"\n-222,\"Data out of range\"\n-222,\"Data out of range\"\n-222,\"Data out of range\"\n-222,\"Data out of range\"\n-222,\"Data out of range\"\n-222,\"Data out of range\"\n-222,\"Data out of range\"\n-222,\"Data out of range\"\n-222,\"Data out of range\"\n-222,\"Data out of range\"\n-222,\"Data out of range\"\n-222,\"Data out of range\"\n-222,\"Data out of range\"\n-222,\"Data out of range\"\n-222,\"Data out of range\"\n-222,\"Data out of range\"\n-222,\"Data out of range\"\n-222,\"Data out of range\"\n-222,\"Data out of range\"\n-222,\"Data out of range\"\n-222,\"Data out of range\"\n-222,\"Data out of range\"\n-222,\"Data out of range\"\n-222,\"Data out of range\"\n-222,\"Data out of range\"\n-222,\"Data out of range\"\n-222,\"Data out of range\"\n-222,\"Data out of range\"\n-222,\"Data out of range\"\n-222,\"Data out of range\"\n-222,\"Data out of range\"\n-222,\"Data out of range\"\n-222,\"Data out of range\"\n-222,\"Data out of range\"\n-222,\"Data out of range\"\n-222,\"Data out of range\"\n-222,\"Data out of range\"\n-222,\"Data out of range\"\n-222,\"Data out of range\"\n-222,\"Data out of range\"\n-222,\"Data out of range\"\n-222,\"Data out of range\"\n-222,\"Data out of range\"\n-222,\"Data out of range\"\n-222,\"Data out of range\"\n-222,\"Data out of range\"\n-222,\"Data out of range\"\n-222,\"Data out of range\"\n-222,\"Data out of range\"\n-222,\"Data out of range\"\n-222,\"Data out of range\"\n-222,\"Data out of range\"\n-222,\"Data out of range\"\n-222,\"Data out of range\"\n-222,\"Data out of range\"\n-222,\"Data out of range\"\n-222,\"Data out of range\"\n-222,\"Data out of range\"\n-222,\"Data out of range\"\n-222,\"Data out of range\"\n-222,\"Data out of range\"\n-222,\"Data out of range\"\n-222,\"Data out of range\"\n-222,\"Data out of range\"\n-222,\"Data out of range\"\n-222,\"Data out of range\"\n-222,\"Data out of range\"\n-222,\"Data out of range\"\n-222,\"Data out of range\"\n-222,\"Data out of range\"\n-222,\"Data out of range\"\n-222,\"Data out of range\"\n-222,\"Data out of range\"\n-222,\"Data out of range\"\n-222,\"Data out of range\"\n-222,\"Data out of range\"\n-222,\"Data out of range\"\n-222,\"Data out of range\"\n-222,\"Data out of range\"\n-222,\"Data out of range\"\n-222,\"Data out of range\"\n-222,\"Data out of range\"\n-222,\"Data out of range\"\n-222,\"Data out of range\"\n-222,\"Data out of range\"\n-222,\"Data out of range\"\n-222,\"Data out of range\"\n-222,\"Data out of range\"\n-222,\"Data out of range\"\n-222,\"Data out of range\"\n-222,\"Data out of range\"\n-222,\"Data out of range\"\n-222,\"Data out of range\"\n-222,\"Data out of range\"\n-222,\"Data out of range\"\n-222,\"Data out of range\"\n-222,\"Data out of range\"\n-222,\"Data out of range\"\n-222,\"Data out of range\"\n-222,\"Data out of range\"\n-222,\"Data out of range\"\n-222,\"Data out of range\"\n-222,\"Data out of range\"\n-222,\"Data out of range\"\n-222,\"Data out of range\"\n-222,\"Data out of range\"\n-222,\"Data out of range\"\n-222,\"Data out of range\"\n-222,\"Data out of range\"\n-222,\"Data out of range\"\n-222,\"Data out of range\"\n-222,\"Data out of range\"\n-222,\"Data out of range\"\n-222,\"Data out of range\"\n-222,\"Data out of range\"\n-222,\"Data out of range\"\n-222,\"Data out of range\"\n-222,\"Data out of range\"\n-222,\"Data out of range\"\n-222,\"Data out of range\"\n-222,\"Data out of range\"\n-222,\"Data out of range\"\n-222,\"Data out of range\"\n-222,\"Data out of range\"\n-222,\"Data out of range\"\n-222,\"Data out of range\"\n-222,\"Data out of range\"\n-222,\"Data out of range\"\n-222,\"Data out of range\"\n-222,\"Data out of range\"\n-222,\"Data out of range\"\n-222,\"Data out of range\"\n-222,\"Data out of range\"\n-222,\"Data out of range\"\n-222,\"Data out of range\"\n-222,\"Data out of range\"\n-222,\"Data out of range\"\n-222,\"Data out of range\"\n-222,\"Data out of range\"\n-222,\"Data out of range\"\n-222,\"Data out of range\"\n-222,\"Data out of range\"\n-222,\"Data out of range\"\n-222,\"Data out of range\"\n-222,\"Data out of range\"\n-222,\"Data out of range\"\n-222,\"Data out of range\"\n-222,\"Data out of range\"\n-222,\"Data out of range\"\n-222,\"Data out of range\"\n-222,\"Data out of range\"\n-222,\"Data out of range\"\n-222,\"Data out of range\"\n-222,\"Data out of range\"\n-222,\"Data out of range\"\n-222,\"Data out of range\"\n-222,\"Data out of range\"\n-222,\"Data out of range\"\n-222,\"Data out of range\"\n-222,\"Data out of range\"\n-222,\"Data out of range\"\n-222,\"Data out of range\"\n-222,\"Data out of range\"\n-222,\"Data out of range\"\n-222,\"Data out of range\"\n-222,\"Data out of range\"\n-222,\"Data out of range\"\n-222,\"Data out of range\"\n-222,\"Data out of range\"\n-222,\"Data out of range\"\n-222,\"Data out of range\"\n-222,\"Data out of range\"\n-222,\"Data out of range\"\n-222,\"Data out of range\"\n-222,\"Data out of range\"\n-222,\"Data out of range\"\n-222,\"Data out of range\"\n-222,\"Data out of range\"\n-222,\"Data out of range\"\n-222,\"Data out of range\"\n-222,\"Data out of range\"\n-222,\"Data out of range\"\n-222,\"Data out of range\"\n-222,\"Data out of range\"\n-222,\"Data out of range\"\n-222,\"Data out of range\"\n-222,\"Data out of range\"\n-222,\"Data out of range\"\n-222,\"Data out of range\"\n-222,\"Data out of range\"\n-222,\"Data out of range\"\n-222,\"Data out of range\"\n-222,\"Data out of range\"\n-222,\"Data out of range\"\n-222,\"Data out of range\"\n-222,\"Data out of range\"\n-222,\"Data out of range\"\n-222,\"Data out of range\"\n-222,\"Data out of range\"\n-222,\"Data out of range\"\n-222,\"Data out of range\"\n-222,\"Data out of range\"\n-222,\"Data out of range\"\n-222,\"Data out of range\"\n-222,\"Data out of range\"\n-222,\"Data out of range\"\n-222,\"Data out of range\"\n-222,\"Data out of range\"\n-222,\"Data out of range\"\n-222,\"Data out of range\"\n-222,\"Data out of range\"\n-222,\"Data out of range\"\n-222,\"Data out of range\"\n-222,\"Data out of range\"\n-222,\"Data out of range\"\n-222,\"Data out of range\"\n-222,\"Data out of range\"\n-222,\"Data out of range\"\n-222,\"Data out of range\"\n-222,\"Data out of range\"\n-222,\"Data out of range\"\n-222,\"Data out of range\"\n-222,\"Data out of range\"\n-222,\"Data out of range\"\n-222,\"Data out of range\"\n-222,\"Data out of range\"\n-222,\"Data out of range\"\n-222,\"Data out of range\"\n-222,\"Data out of range\"\n-222,\"Data out of range\"\n-222,\"Data out of range\"\n-222,\"Data out of range\"\n-222,\"Data out of range\"\n-222,\"Data out of range\"\n-222,\"Data out of range\"\n-222,\"Data out of range\"\n-222,\"Data out of range\"\n-222,\"Data out of range\"\n-222,\"Data out of range\"\n-222,\"Data out of range\"\n-222,\"Data out of range\"\n-222,\"Data out of range\"\n-222,\"Data out of range\"\n-222,\"Data out of range\"\n-222,\"Data out of range\"\n-222,\"Data out of range\"\n-222,\"Data out of range\"\n-222,\"Data out of range\"\n-222,\"Data out of range\"\n-222,\"Data out of range\"\n-222,\"Data out of range\"\n-222,\"Data out of range\"\n-222,\"Data out of range\"\n-222,\"Data out of range\"\n-222,\"Data out of range\"\n-222,\"Data out of range\"\n-222,\"Data out of range\"\n-222,\"Data out of range\"\n-222,\"Data out of range\"\n-222,\"Data out of range\"\n-222,\"Data out of range\"\n-222,\"Data out of range\"\n-222,\"Data out of range\"\n-222,\"Data out of range\"\n-222,\"Data out of range\"\n-222,\"Data out of range\"\n-222,\"Data out of range\"\n-222,\"Data out of range\"\n-222,\"Data out of range\"\n-222,\"Data out of range\"\n-222,\"Data out of range\"\n-222,\"Data out of range\"\n-222,\"Data out of range\"\n-222,\"Data out of range\"\n-222,\"Data out of range\"\n-222,\"Data out of range\"\n-222,\"Data out of range\"\n-222,\"Data out of range\"\n-222,\"Data out of range\"\n-222,\"Data out of range\"\n-222,\"Data out of range\"\n-222,\"Data out of range\"\n-222,\"Data out of range\"\n-222,\"Data out of range\"\n-222,\"Data out of range\"\n-222,\"Data out of range\"\n-222,\"Data out of range\"\n-222,\"Data out of range\"\n-222,\"Data out of range\"\n-222,\"Data out of range\"\n-222,\"Data out of range\"\n-222,\"Data out of range\"\n-222,\"Data out of range\"\n-222,\"Data out of range\"\n-222,\"Data out of range\"\n-222,\"Data out of range\"\n-222,\"Data out of range\"\n-222,\"Data out of range\"\n-222,\"Data out of range\"\n-222,\"Data out of range\"\n-222,\"Data out of range\"\n-222,\"Data out of range\"\n-222,\"Data out of range\"\n-222,\"Data out of range\"\n-222,\"Data out of range\"\n-222,\"Data out of range\"\n-222,\"Data out of range\"\n-222,\"Data out of range\"\n-222,\"Data out of range\"\n-222,\"Data out of range\"\n-222,\"Data out of range\"\n-222,\"Data out of range\"\n-222,\"Data out of range\"\n-222,\"Data out of range\"\n-222,\"Data out of range\"\n-222,\"Data out of range\"\n-222,\"Data out of range\"\n-222,\"Data out of range\"\n-222,\"Data out of range\"\n-222,\"Data out of range\"\n-222,\"Data out of range\"\n-222,\"Data out of range\"\n-222,\"Data out of range\"\n-222,\"Data out of range\"\n-222,\"Data out of range\"\n-222,\"Data out of range\"\n-222,\"Data out of range\"\n-222,\"Data out of range\"\n-222,\"Data out of range\"\n-222,\"Data out of range\"\n-222,\"Data out of range\"\n-222,\"Data out of range\"\n-222,\"Data out of range\"\n-222,\"Data out of range\"\n-222,\"Data out of range\"\n-222,\"Data out of range\"\n-222,\"Data out of range\"\n-222,\"Data out of range\"\n-222,\"Data out of range\"\n-222,\"Data out of range\"\n-222,\"Data out of range\"\n-222,\"Data out of range\"\n-222,\"Data out of range\"\n-222,\"Data out of range\"\n-222,\"Data out of range\"\n-222,\"Data out of range\"\n-222,\"Data out of range\"\n-222,\"Data out of range\"\n-222,\"Data out of range\"\n-222,\"Data out of range\"\n-222,\"Data out of range\"\n-222,\"Data out of range\"\n-222,\"Data out of range\"\n-222,\"Data out of range\"\n-222,\"Data out of range\"\n-222,\"Data out of range\"\n-222,\"Data out of range\"\n-222,\"Data out of range\"\n-222,\"Data out of range\"\n-222,\"Data out of range\"\n-222,\"Data out of range\"\n-222,\"Data out of range\"\n-222,\"Data out of range\"\n-222,\"Data out of range\"\n-222,\"Data out of range\"\n-222,\"Data out of range\"\n-222,\"Data out of range\"\n-222,\"Data out of range\"\n-222,\"Data out of range\"\n-222,\"Data out of range\"\n-222,\"Data out of range\"\n-222,\"Data out of range\"\n-222,\"Data out of range\"\n-222,\"Data out of range\"\n-222,\"Data out of range\"\n-222,\"Data out of range\"\n-222,\"Data out of range\"\n-222,\"Data out of range\"\n-222,\"Data out of range\"\n-222,\"Data out of range\"\n-222,\"Data out of range\"\n-222,\"Data out of range\"\n-222,\"Data out of range\"\n-222,\"Data out of range\"\n-222,\"Data out of range\"\n-222,\"Data out of range\"\n-222,\"Data out of range\"\n-222,\"Data out of range\"\n-222,\"Data out of range\"\n-222,\"Data out of range\"\n-222,\"Data out of range\"\n-222,\"Data out of range\"\n-222,\"Data out of range\"\n-222,\"Data out of range\"\n-222,\"Data out of range\"\n-222,\"Data out of range\"\n-222,\"Data out of range\"\n-222,\"Data out of range\"\n-222,\"Data out of range\"\n-222,\"Data out of range\"\n-222,\"Data out of range\"\n-222,\"Data out of range\"\n-222,\"Data out of range\"\n-222,\"Data out of range\"\n-222,\"Data out of range\"\n-222,\"Data out of range\"\n-222,\"Data out of range\"\n-222,\"Data out of range\"\n-222,\"Data out of range\"\n-222,\"Data out of range\"\n-222,\"Data out of range\"\n-222,\"Data out of range\"\n-222,\"Data out of range\"\n-222,\"Data out of range\"\n-222,\"Data out of range\"\n-222,\"Data out of range\"\n-222,\"Data out of range\"\n-222,\"Data out of range\"\n-222,\"Data out of range\"\n-222,\"Data out of range\"\n-222,\"Data out of range\"\n-222,\"Data out of range\"\n-222,\"Data out of range\"\n-222,\"Data out of range\"\n-222,\"Data out of range\"\n-222,\"Data out of range\"\n-222,\"Data out of range\"\n-222,\"Data out of range\"\n-222,\"Data out of range\"\n-222,\"Data out of range\"\n-222,\"Data out of range\"\n-222,\"Data out of range\"\n-222,\"Data out of range\"\n-222,\"Data out of range\"\n-222,\"Data out of range\"\n-222,\"Data out of range\"\n-222,\"Data out of range\"\n-222,\"Data out of range\"\n-222,\"Data out of range\"\n-222,\"Data out of range\"\n-222,\"Data out of range\"\n-222,\"Data out of range\"\n-222,\"Data out of range\"\n-222,\"Data out of range\"\n-222,\"Data out of range\"\n-222,\"Data out of range\"\n-222,\"Data out of range\"\n-222,\"Data out of range\"\n-222,\"Data out of range\"\n-222,\"Data out of range\"\n-222,\"Data out of range\"\n-222,\"Data out of range\"\n-222,\"Data out of range\"\n-222,\"Data out of range\"\n-222,\"Data out of range\"\n-222,\"Data out of range\"\n-222,\"Data out of range\"\n-222,\"Data out of range\"\n-222,\"Data out of range\"\n-222,\"Data out of range\"\n-222,\"Data out of range\"\n-222,\"Data out of range\"\n-222,\"Data out of range\"\n-222,\"Data out of range\"\n-222,\"Data out of range\"\n-222,\"Data out of range\"\n-222,\"Data out of range\"\n-222,\"Data out of range\"\n-222,\"Data out of range\"\n-222,\"Data out of range\"\n-222,\"Data out of range\"\n-222,\"Data out of range\"\n-222,\"Data out of range\"\n-222,\"Data out of range\"\n-222,\"Data out of range\"\n-222,\"Data out of range\"\n-222,\"Data out of range\"\n-222,\"Data out of range\"\n-222,\"Data out of range\"\n-222,\"Data out of range\"\n-222,\"Data out of range\"\n-222,\"Data out of range\"\n-222,\"Data out of range\"\n-222,\"Data out of range\"\n-222,\"Data out of range\"\n-222,\"Data out of range\"\n-222,\"Data out of range\"\n-222,\"Data out of range\"\n-222,\"Data out of range\"\n-222,\"Data out of range\"\n-222,\"Data out of range\"\n-222,\"Data out of range\"\n-222,\"Data out of range\"\n-222,\"Data out of range\"\n-222,\"Data out of range\"\n-222,\"Data out of range\"\n-222,\"Data out of range\"\n-222,\"Data out of range\"\n-222,\"Data out of range\"\n-222,\"Data out of range\"\n-222,\"Data out of range\"\n-222,\"Data out of range\"\n-222,\"Data out of range\"\n-222,\"Data out of range\"\n-222,\"Data out of range\"\n-222,\"Data out of range\"\n-222,\"Data out of range\"\n-222,\"Data out of range\"\n-222,\"Data out of range\"\n-222,\"Data out of range\"\n-222,\"Data out of range\"\n-222,\"Data out of range\"\n-222,\"Data out of range\"\n-222,\"Data out of range\"\n-222,\"Data out of range\"\n-222,\"Data out of range\"\n-222,\"Data out of range\"\n-222,\"Data out of range\"\n-222,\"Data out of range\"\n-222,\"Data out of range\"\n-222,\"Data out of range\"\n-222,\"Data out of range\"\n-222,\"Data out of range\"\n-222,\"Data out of range\"\n-222,\"Data out of range\"\n-222,\"Data out of range\"\n-222,\"Data out of range\"\n-222,\"Data out of range\"\n-222,\"Data out of range\"\n-222,\"Data out of range\"\n-222,\"Data out of range\"\n-222,\"Data out of range\"\n-222,\"Data out of range\"\n-222,\"Data out of range\"\n-222,\"Data out of range\"\n-222,\"Data out of range\"\n-222,\"Data out of range\"\n-222,\"Data out of range\"\n-222,\"Data out of range\"\n-222,\"Data out of range\"\n-222,\"Data out of range\"\n-222,\"Data out of range\"\n-222,\"Data out of range\"\n-222,\"Data out of range\"\n-222,\"Data out of range\"\n-222,\"Data out of range\"\n-222,\"Data out of range\"\n-222,\"Data out of range\"\n-222,\"Data out of range\"\n-222,\"Data out of range\"\n-222,\"Data out of range\"\n-222,\"Data out of range\"\n-222,\"Data out of range\"\n-222,\"Data out of range\"\n-222,\"Data out of range\"\n-222,\"Data out of range\"\n-222,\"Data out of range\"\n-222,\"Data out of range\"\n-222,\"Data out of range\"\n-222,\"Data out of range\"\n-222,\"Data out of range\"\n-222,\"Data out of range\"\n-222,\"Data out of range\"\n-222,\"Data out of range\"\n-222,\"Data out of range\"\n-222,\"Data out of range\"\n-222,\"Data out of range\"\n-222,\"Data out of range\"\n-222,\"Data out of range\"\n-222,\"Data out of range\"\n-222,\"Data out of range\"\n-222,\"Data out of range\"\n-222,\"Data out of range\"\n-222,\"Data out of range\"\n-222,\"Data out of range\"\n-222,\"Data out of range\"\n-222,\"Data out of range\"\n-222,\"Data out of range\"\n-222,\"Data out of range\"\n-222,\"Data out of range\"\n-222,\"Data out of range\"\n-222,\"Data out of range\"\n-222,\"Data out of range\"\n-222,\"Data out of range\"\n-222,\"Data out of range\"\n-222,\"Data out of range\"\n-222,\"Data out of range\"\n-222,\"Data out of range\"\n-222,\"Data out of range\"\n-222,\"Data out of range\"\n-222,\"Data out of range\"\n-222,\"Data out of range\"\n-222,\"Data out of range\"\n-222,\"Data out of range\"\n-222,\"Data out of range\"\n-222,\"Data out of range\"\n-222,\"Data out of range\"\n-222,\"Data out of range\"\n-222,\"Data out of range\"\n-222,\"Data out of range\"\n-222,\"Data out of range\"\n-222,\"Data out of range\"\n-222,\"Data out of range\"\n-222,\"Data out of range\"\n-222,\"Data out of range\"\n-222,\"Data out of range\"\n-222,\"Data out of range\"\n-222,\"Data out of range\"\n-222,\"Data out of range\"\n-222,\"Data out of range\"\n-222,\"Data out of range\"\n-222,\"Data out of range\"\n-222,\"Data out of range\"\n-222,\"Data out of range\"\n-222,\"Data out of range\"\n-222,\"Data out of range\"\n-222,\"Data out of range\"\n-222,\"Data out of range\"\n-222,\"Data out of range\"\n-222,\"Data out of range\"\n-222,\"Data out of range\"\n-222,\"Data out of range\"\n-222,\"Data out of range\"\n-222,\"Data out of range\"\n-222,\"Data out of range\"\n-222,\"Data out of range\"\n-222,\"Data out of range\"\n-222,\"Data out of range\"\n-222,\"Data out of range\"\n-222,\"Data out of range\"\n-222,\"Data out of range\"\n-222,\"Data out of range\"\n-222,\"Data out of range\"\n-222,\"Data out of range\"\n-222,\"Data out of range\"\n-222,\"Data out of range\"\n-222,\"Data out of range\"\n-222,\"Data out of range\"\n-222,\"Data out of range\"\n-222,\"Data out of range\"\n-222,\"Data out of range\"\n-222,\"Data out of range\"\n-222,\"Data out of range\"\n-222,\"Data out of range\"\n-222,\"Data out of range\"\n-222,\"Data out of range\"\n-222,\"Data out of range\"\n-222,\"Data out of range\"\n-222,\"Data out of range\"\n-222,\"Data out of range\"\n-222,\"Data out of range\"\n-222,\"Data out of range\"\n-222,\"Data out of range\"\n-222,\"Data out of range\"\n-222,\"Data out of range\"\n-222,\"Data out of range\"\n-222,\"Data out of range\"\n-222,\"Data out of range\"\n-222,\"Data out of range\"\n-222,\"Data out of range\"\n-222,\"Data out of range\"\n-222,\"Data out of range\"\n-222,\"Data out of range\"\n-222,\"Data out of range\"\n-222,\"Data out of range\"\n-222,\"Data out of range\"\n-222,\"Data out of range\"\n-222,\"Data out of range\"\n-222,\"Data out of range\"\n-222,\"Data out of range\"\n-222,\"Data out of range\"\n-222,\"Data out of range\"\n-222,\"Data out of range\"\n-222,\"Data out of range\"\n-222,\"Data out of range\"\n-222,\"Data out of range\"\n-222,\"Data out of range\"\n-222,\"Data out of range\"\n-222,\"Data out of range\"\n-222,\"Data out of range\"\n-222,\"Data out of range\"\n-222,\"Data out of range\"\n-222,\"Data out of range\"\n-222,\"Data out of range\"\n-222,\"Data out of range\"\n-222,\"Data out of range\"\n-222,\"Data out of range\"\n-222,\"Data out of range\"\n-222,\"Data out of range\"\n-222,\"Data out of range\"\n-222,\"Data out of range\"\n-222,\"Data out of range\"\n-222,\"Data out of range\"\n-222,\"Data out of range\"\n-222,\"Data out of range\"\n-222,\"Data out of range\"\n-222,\"Data out of range\"\n-222,\"Data out of range\"\n-222,\"Data out of range\"\n-222,\"Data out of range\"\n-222,\"Data out of range\"\n-222,\"Data out of range\"\n-222,\"Data out of range\"\n-222,\"Data out of range\"\n-222,\"Data out of range\"\n-222,\"Data out of range\"\n-222,\"Data out of range\"\n-222,\"Data out of range\"\n-222,\"Data out of range\"\n-222,\"Data out of range\"\n-222,\"Data out of range\"\n-222,\"Data out of range\"\n-222,\"Data out of range\"\n-222,\"Data out of range\"\n-222,\"Data out of range\"\n-222,\"Data out of range\"\n-222,\"Data out of range\"\n-222,\"Data out of range\"\n-222,\"Data out of range\"\n-222,\"Data out of range\"\n-222,\"Data out of range\"\n-222,\"Data out of range\"\n-222,\"Data out of range\"\n-222,\"Data out of range\"\n-222,\"Data out of range\"\n-222,\"Data out of range\"\n-222,\"Data out of range\"\n-222,\"Data out of range\"\n-222,\"Data out of range\"\n-222,\"Data out of range\"\n-222,\"Data out of range\"\n-222,\"Data out of range\"\n-222,\"Data out of range\"\n-222,\"Data out of range\"\n-222,\"Data out of range\"\n-222,\"Data out of range\"\n-222,\"Data out of range\"\n-222,\"Data out of range\"\n-222,\"Data out of range\"\n-222,\"Data out of range\"\n-222,\"Data out of range\"\n-222,\"Data out of range\"\n-222,\"Data out of range\"\n-222,\"Data out of range\"\n-222,\"Data out of range\"\n-222,\"Data out of range\"\n-222,\"Data out of range\"\n-222,\"Data out of range\"\n-222,\"Data out of range\"\n-222,\"Data out of range\"\n-222,\"Data out of range\"\n-222,\"Data out of range\"\n-222,\"Data out of range\"\n-222,\"Data out of range\"\n-222,\"Data out of range\"\n-222,\"Data out of range\"\n-222,\"Data out of range\"\n-222,\"Data out of range\"\n-222,\"Data out of range\"\n-222,\"Data out of range\"\n-222,\"Data out of range\"\n-222,\"Data out of range\"\n-222,\"Data out of range\"\n-222,\"Data out of range\"\n-222,\"Data out of range\"\n-222,\"Data out of range\"\n-222,\"Data out of range\"\n-222,\"Data out of range\"\n-222,\"Data out of range\"\n-222,\"Data out of range\"\n-222,\"Data out of range\"\n-222,\"Data out of range\"\n-222,\"Data out of range\"\n-222,\"Data out of range\"\n-222,\"Data out of range\"\n-222,\"Data out of range\"\n-222,\"Data out of range\"\n-222,\"Data out of range\"\n-222,\"Data out of range\"\n-222,\"Data out of range\"\n-222,\"Data out of range\"\n-222,\"Data out of range\"\n-222,\"Data out of range\"\n-222,\"Data out of range\"\n-222,\"Data out of range\"\n-222,\"Data out of range\"\n-222,\"Data out of range\"\n-222,\"Data out of range\"\n-222,\"Data out of range\"\n-222,\"Data out of range\"\n-222,\"Data out of range\"\n-222,\"Data out of range\"\n-222,\"Data out of range\"\n-222,\"Data out of range\"\n-222,\"Data out of range\"\n-222,\"Data out of range\"\n-222,\"Data out of range\"\n-222,\"Data out of range\"\n-222,\"Data out of range\"\n-222,\"Data out of range\"\n-222,\"Data out of range\"\n-222,\"Data out of range\"\n-222,\"Data out of range\"\n-222,\"Data out of range\"\n-222,\"Data out of range\"\n-222,\"Data out of range\"\n-222,\"Data out of range\"\n-222,\"Data out of range\"\n-222,\"Data out of range\"\n-222,\"Data out of range\"\n-222,\"Data out of range\"\n-222,\"Data out of range\"\n-222,\"Data out of range\"\n-222,\"Data out of range\"\n-222,\"Data out of range\"\n-222,\"Data out of range\"\n-222,\"Data out of range\"\n-222,\"Data out of range\"\n-222,\"Data out of range\"\n-222,\"Data out of range\"\n-222,\"Data out of range\"\n-222,\"Data out of range\"\n-222,\"Data out of range\"\n-222,\"Data out of range\"\n-222,\"Data out of range\"\n-222,\"Data out of range\"\n-222,\"Data out of range\"\n-222,\"Data out of range\"\n-222,\"Data out of range\"\n-222,\"Data out of range\"\n-222,\"Data out of range\"\n-222,\"Data out of range\"\n-222,\"Data out of range\"\n-222,\"Data out of range\"\n-222,\"Data out of range\"\n-222,\"Data out of range\"\n-222,\"Data out of range\"\n-222,\"Data out of range\"\n-222,\"Data out of range\"\n-222,\"Data out of range\"\n-222,\"Data out of range\"\n-222,\"Data out of range\"\n-222,\"Data out of range\"\n-222,\"Data out of range\"\n-222,\"Data out of range\"\n-222,\"Data out of range\"\n-222,\"Data out of range\"\n-222,\"Data out of range\"\n-222,\"Data out of range\"\n-222,\"Data out of range\"\n-222,\"Data out of range\"\n-222,\"Data out of range\"\n-222,\"Data out of range\"\n-222,\"Data out of range\"\n-222,\"Data out of range\"\n-222,\"Data out of range\"\n-222,\"Data out of range\"\n-222,\"Data out of range\"\n-222,\"Data out of range\"\n-222,\"Data out of range\"\n-222,\"Data out of range\"\n-222,\"Data out of range\"\n-222,\"Data out of range\"\n-222,\"Data out of range\"\n-222,\"Data out of range\"\n-222,\"Data out of range\"\n-222,\"Data out of range\"\n-222,\"Data out of range\"\n-222,\"Data out of range\"\n-222,\"Data out of range\"\n-222,\"Data out of range\"\n-222,\"Data out of range\"\n-222,\"Data out of range\"\n-222,\"Data out of range\"\n-222,\"Data out of range\"\n-222,\"Data out of range\"\n-222,\"Data out of range\"\n-222,\"Data out of range\"\n-222,\"Data out of range\"\n-222,\"Data out of range\"\n-222,\"Data out of range\"\n-222,\"Data out of range\"\n-222,\"Data out of range\"\n-222,\"Data out of range\"\n-222,\"Data out of range\"\n-222,\"Data out of range\"\n-222,\"Data out of range\"\n-222,\"Data out of range\"\n-222,\"Data out of range\"\n-222,\"Data out of range\"\n-222,\"Data out of range\"\n-222,\"Data out of range\"\n-222,\"Data out of range\"\n-222,\"Data out of range\"\n-222,\"Data out of range\"\n-222,\"Data out of range\"\n-222,\"Data out of range\"\n-222,\"Data out of range\"\n-222,\"Data out of range\"\n-222,\"Data out of range\"\n-222,\"Data out of range\"\n-222,\"Data out of range\"\n-222,\"Data out of range\"\n-222,\"Data out of range\"\n-222,\"Data out of range\"\n-222,\"Data out of range\"\n-222,\"Data out of range\"\n-222,\"Data out of range\"\n-222,\"Data out of range\"\n-222,\"Data out of range\"\n-222,\"Data out of range\"\n-222,\"Data out of range\"\n-222,\"Data out of range\"\n-222,\"Data out of range\"\n-222,\"Data out of range\"\n-222,\"Data out of range\"\n-222,\"Data out of range\"\n-222,\"Data out of range\"\n-222,\"Data out of range\"\n-222,\"Data out of range\"\n-222,\"Data out of range\"\n-222,\"Data out of range\"\n-222,\"Data out of range\"\n-222,\"Data out of range\"\n-222,\"Data out of range\"\n-222,\"Data out of range\"\n-222,\"Data out of range\"\n-222,\"Data out of range\"\n-222,\"Data out of range\"\n-222,\"Data out of range\"\n-222,\"Data out of range\"\n-222,\"Data out of range\"\n-222,\"Data out of range\"\n-222,\"Data out of range\"\n-222,\"Data out of range\"\n-222,\"Data out of range\"\n-222,\"Data out of range\"\n-222,\"Data out of range\"\n-222,\"Data out of range\"\n-222,\"Data out of range\"\n-222,\"Data out of range\"\n-222,\"Data out of range\"\n-222,\"Data out of range\"\n-222,\"Data out of range\"\n-222,\"Data out of range\"\n-222,\"Data out of range\"\n-222,\"Data out of range\"\n-222,\"Data out of range\"\n-222,\"Data out of range\"\n-222,\"Data out of range\"\n-222,\"Data out of range\"\n-222,\"Data out of range\"\n-222,\"Data out of range\"\n-222,\"Data out of range\"\n-222,\"Data out of range\"\n-222,\"Data out of range\"\n-222,\"Data out of range\"\n-222,\"Data out of range\"\n-222,\"Data out of range\"\n-222,\"Data out of range\"\n-222,\"Data out of range\"\n-222,\"Data out of range\"\n-222,\"Data out of range\"\n-222,\"Data out of range\"\n-222,\"Data out of range\"\n-222,\"Data out of range\"\n-222,\"Data out of range\"\n-222,\"Data out of range\"\n-222,\"Data out of range\"\n-222,\"Data out of range\"\n-222,\"Data out of range\"\n-222,\"Data out of range\"\n-222,\"Data out of range\"\n-222,\"Data out of range\"\n-222,\"Data out of range\"\n-222,\"Data out of range\"\n-222,\"Data out of range\"\n-222,\"Data out of range\"\n-222,\"Data out of range\"\n-222,\"Data out of range\"\n-222,\"Data out of range\"\n-222,\"Data out of range\"\n-222,\"Data out of range\"\n-222,\"Data out of range\"\n-222,\"Data out of range\"\n-222,\"Data out of range\"\n-222,\"Data out of range\"\n-222,\"Data out of range\"\n-222,\"Data out of range\"\n-222,\"Data out of range\"\n-222,\"Data out of range\"\n-222,\"Data out of range\"\n-222,\"Data out of range\"\n-222,\"Data out of range\"\n-222,\"Data out of range\"\n-222,\"Data out of range\"\n-222,\"Data out of range\"\n-222,\"Data out of range\"\n-222,\"Data out of range\"\n-222,\"Data out of range\"\n-222,\"Data out of range\"\n-222,\"Data out of range\"\n-222,\"Data out of range\"\n-222,\"Data out of range\"\n-222,\"Data out of range\"\n-222,\"Data out of range\"\n-222,\"Data out of range\"\n-222,\"Data out of range\"\n-222,\"Data out of range\"\n-222,\"Data out of range\"\n-222,\"Data out of range\"\n-222,\"Data out of range\"\n-222,\"Data out of range\"\n-222,\"Data out of range\"\n-222,\"Data out of range\"\n-222,\"Data out of range\"\n-222,\"Data out of range\"\n-222,\"Data out of range\"\n-222,\"Data out of range\"\n-222,\"Data out of range\"\n-222,\"Data out of range\"\n-222,\"Data out of range\"\n-222,\"Data out of range\"\n-222,\"Data out of range\"\n-222,\"Data out of range\"\n-222,\"Data out of range\"\n-222,\"Data out of range\"\n-222,\"Data out of range\"\n-222,\"Data out of range\"\n-222,\"Data out of range\"\n-222,\"Data out of range\"\n-222,\"Data out of range\"\n-222,\"Data out of range\"\n-222,\"Data out of range\"\n-222,\"Data out of range\"\n-222,\"Data out of range\"\n-222,\"Data out of range\"\n-222,\"Data out of range\"\n-222,\"Data out of range\"\n-222,\"Data out of range\"\n-222,\"Data out of range\"\n-222,\"Data out of range\"\n-222,\"Data out of range\"\n-222,\"Data out of range\"\n-222,\"Data out of range\"\n-222,\"Data out of range\"\n-222,\"Data out of range\"\n-222,\"Data out of range\"\n-222,\"Data out of range\"\n-222,\"Data out of range\"\n-222,\"Data out of range\"\n-222,\"Data out of range\"\n-222,\"Data out of range\"\n-222,\"Data out of range\"\n-222,\"Data out of range\"\n-222,\"Data out of range\"\n-222,\"Data out of range\"\n-222,\"Data out of range\"\n-222,\"Data out of range\"\n-222,\"Data out of range\"\n-222,\"Data out of range\"\n-222,\"Data out of range\"\n-222,\"Data out of range\"\n-222,\"Data out of range\"\n-222,\"Data out of range\"\n-222,\"Data out of range\"\n-222,\"Data out of range\"\n-222,\"Data out of range\"\n-222,\"Data out of range\"\n-222,\"Data out of range\"\n-222,\"Data out of range\"\n-222,\"Data out of range\"\n-222,\"Data out of range\"\n-222,\"Data out of range\"\n-222,\"Data out of range\"\n-222,\"Data out of range\"\n-222,\"Data out of range\"\n-222,\"Data out of range\"\n-222,\"Data out of range\"\n-222,\"Data out of range\"\n-222,\"Data out of range\"\n-222,\"Data out of range\"\n-222,\"Data out of range\"\n-222,\"Data out of range\"\n-222,\"Data out of range\"\n-222,\"Data out of range\"\n-222,\"Data out of range\"\n-222,\"Data out of range\"\n-222,\"Data out of range\"\n-222,\"Data out of range\"\n-222,\"Data out of range\"\n-222,\"Data out of range\"\n-222,\"Data out of range\"\n-222,\"Data out of range\"\n-222,\"Data out of range\"\n-222,\"Data out of range\"\n-222,\"Data out of range\"\n-222,\"Data out of range\"\n-222,\"Data out of range\"\n-222,\"Data out of range\"\n-222,\"Data out of range\"\n-222,\"Data out of range\"\n-222,\"Data out of range\"\n-222,\"Data out of range\"\n-222,\"Data out of range\"\n-222,\"Data out of range\"\n-222,\"Data out of range\"\n-222,\"Data out of range\"\n-222,\"Data out of range\"\n-222,\"Data out of range\"\n-222,\"Data out of range\"\n-222,\"Data out of range\"\n-222,\"Data out of range\"\n-222,\"Data out of range\"\n-222,\"Data out of range\"\n-222,\"Data out of range\"\n-222,\"Data out of range\"\n-222,\"Data out of range\"\n-222,\"Data out of range\"\n-222,\"Data out of range\"\n-222,\"Data out of range\"\n-222,\"Data out of range\"\n-222,\"Data out of range\"\n-222,\"Data out of range\"\n-222,\"Data out of range\"\n-222,\"Data out of range\"\n-222,\"Data out of range\"\n-222,\"Data out of range\"\n-222,\"Data out of range\"\n-222,\"Data out of range\"\n-222,\"Data out of range\"\n-222,\"Data out of range\"\n-222,\"Data out of range\"\n"
  out "AUTO?":bool
  out "Zero Value":dbl format="%#.3p"
  out "Rng":string
  in  "Range":i16=1 min=1 max=6 step=1
  in  "Mono Port":refnum<visa-resource-name>="COM10"
  out "IDN String":string="Thorlabs,PM100USB,P2000362,1.3.0\n"
  out "Sensor SN":string="10061433"
  out "Sensor Name":string="S120C"
  out "Reply":string=" 0.000 nm  ok\r\n" caption="Mono Response"
  # "Range Settings"
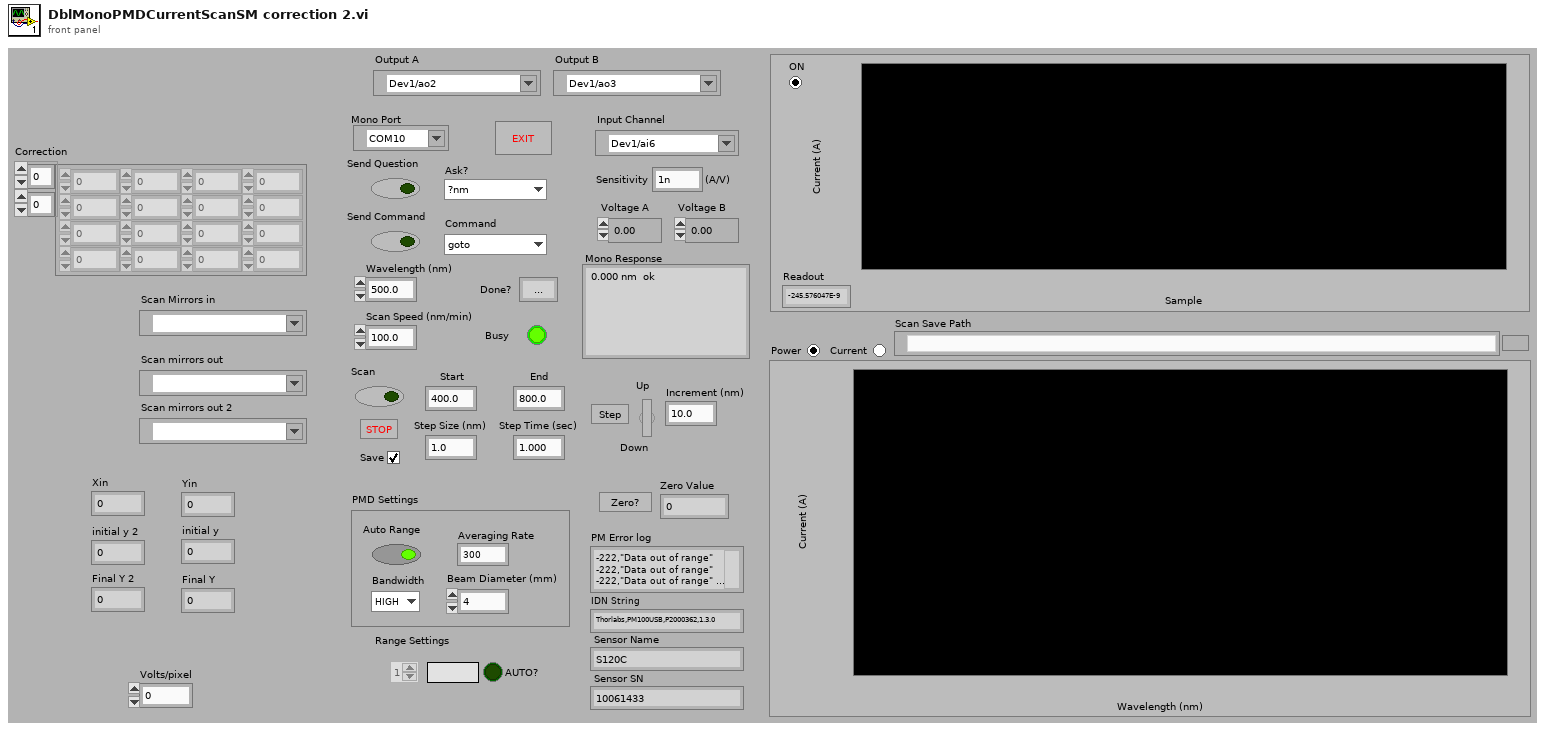
[diagram p1: front panel]
types:
  T1 = cluster{"Beam Diameter (mm)":dbl, "BWIn":u16, "Averaging Rate":i32, "Auto Range":bool}
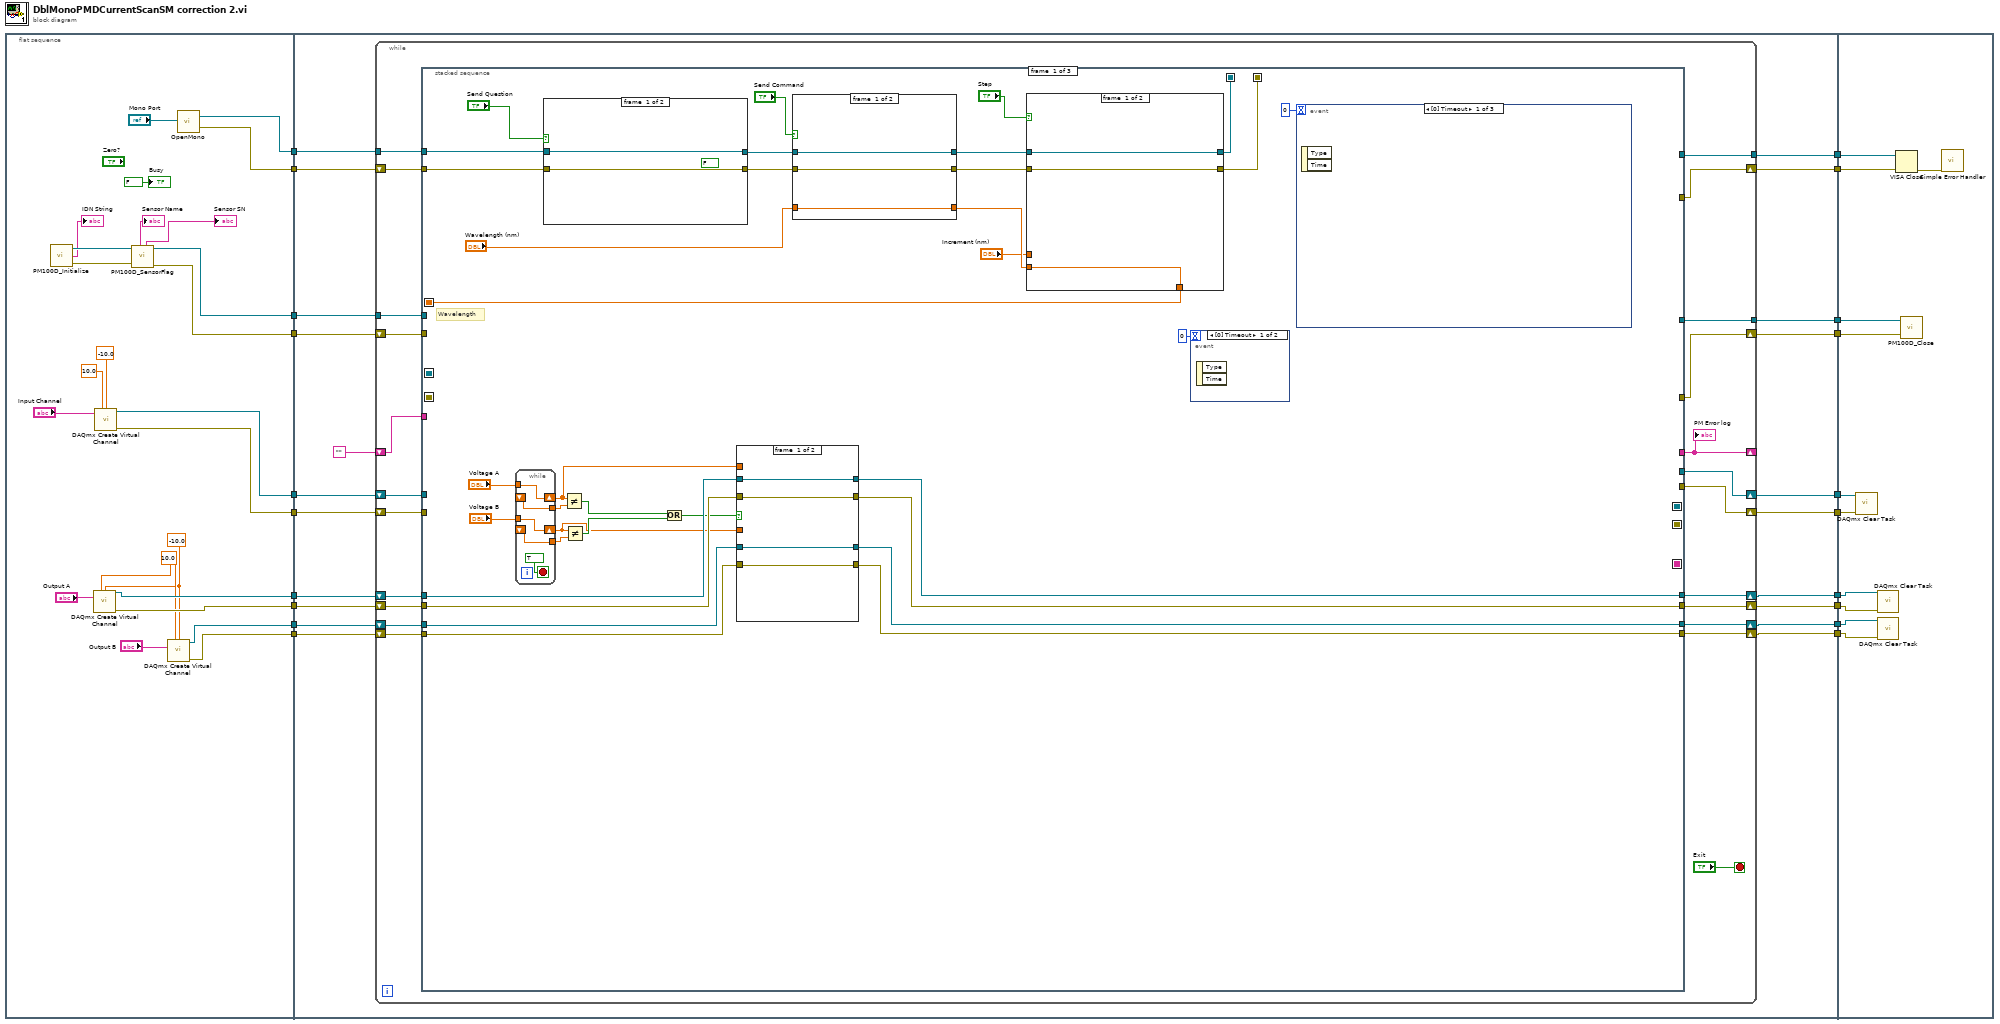
[diagram p0: block diagram]
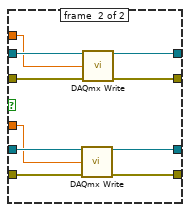
[diagram p2: hidden frame]
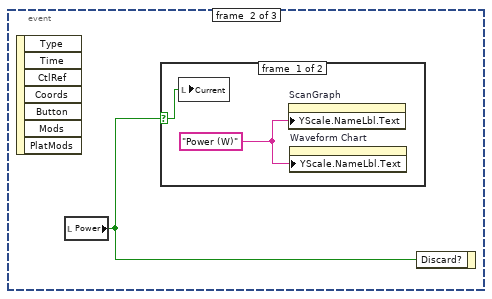
[diagram p3: hidden frame]
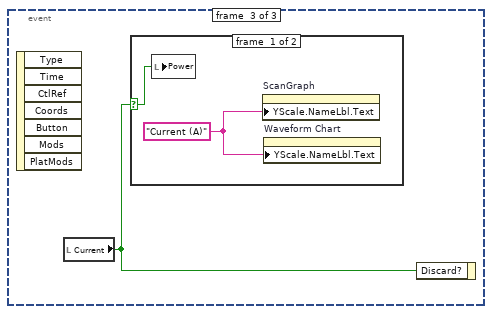
[diagram p5: hidden frame]
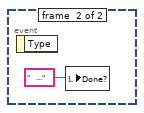
[diagram p7: hidden frame]
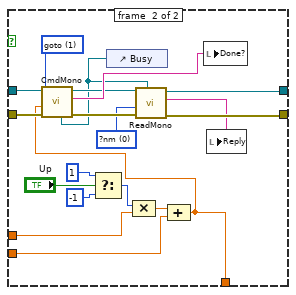
[diagram p8: hidden frame]
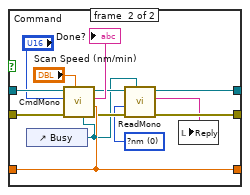
[diagram p9: hidden frame]
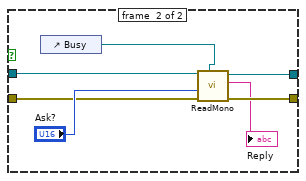
[diagram p10: hidden frame]
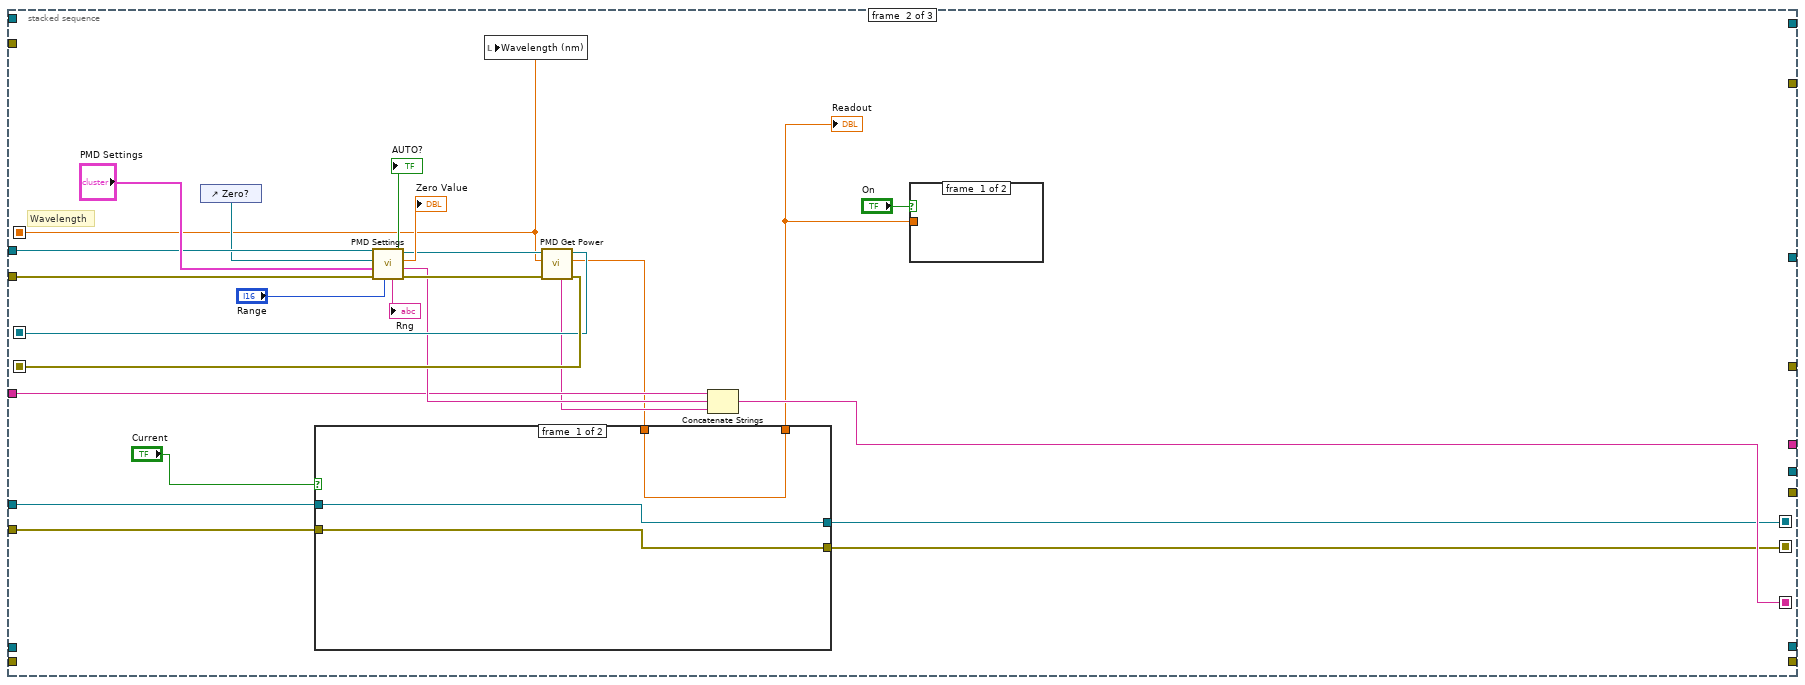
[diagram p11: hidden frame]
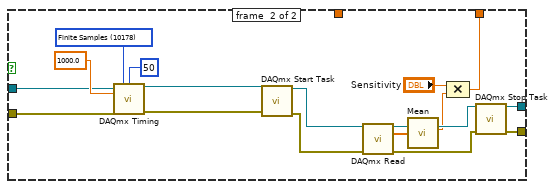
[diagram p12: hidden frame]
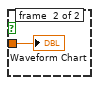
[diagram p13: hidden frame]
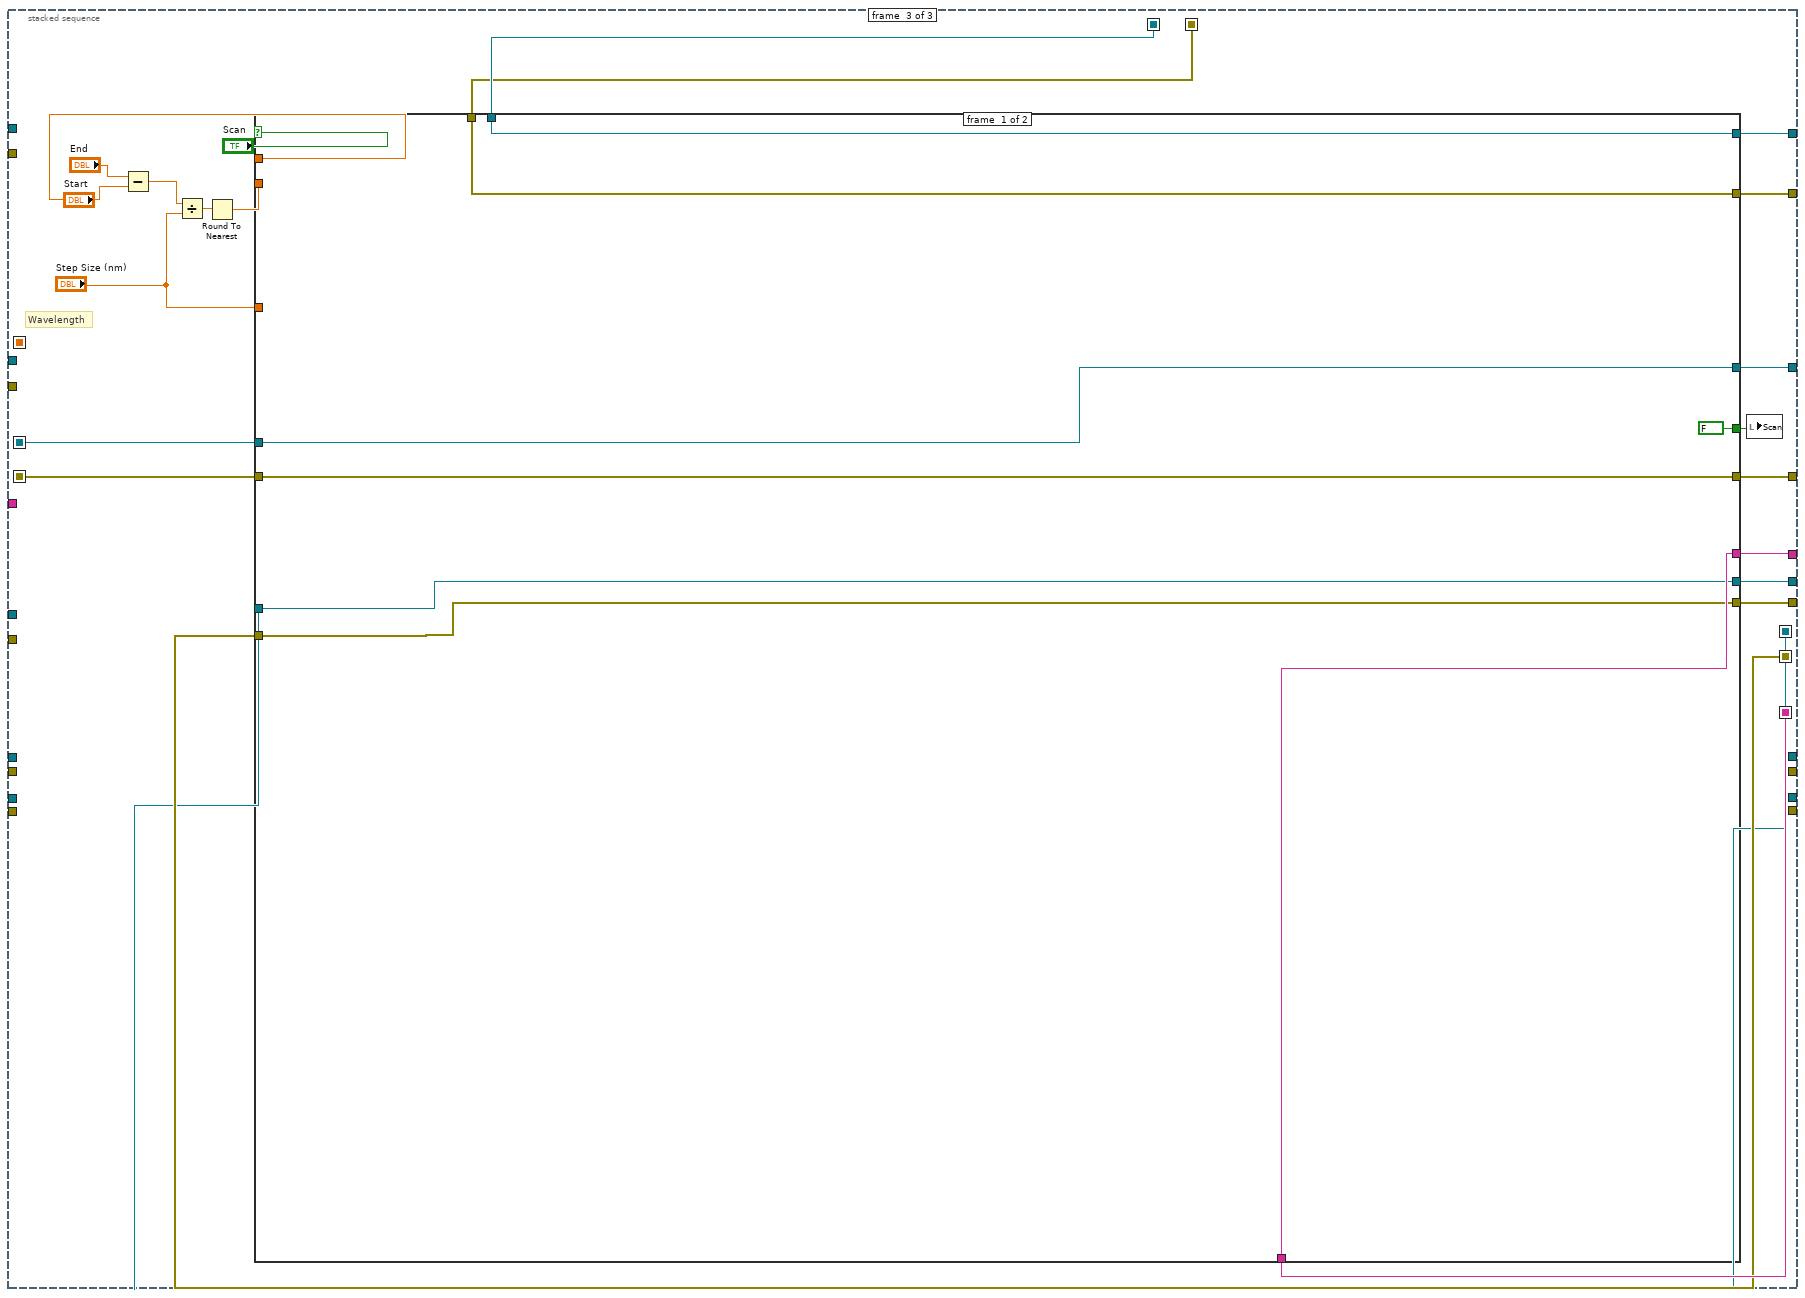
[diagram p14: hidden frame]
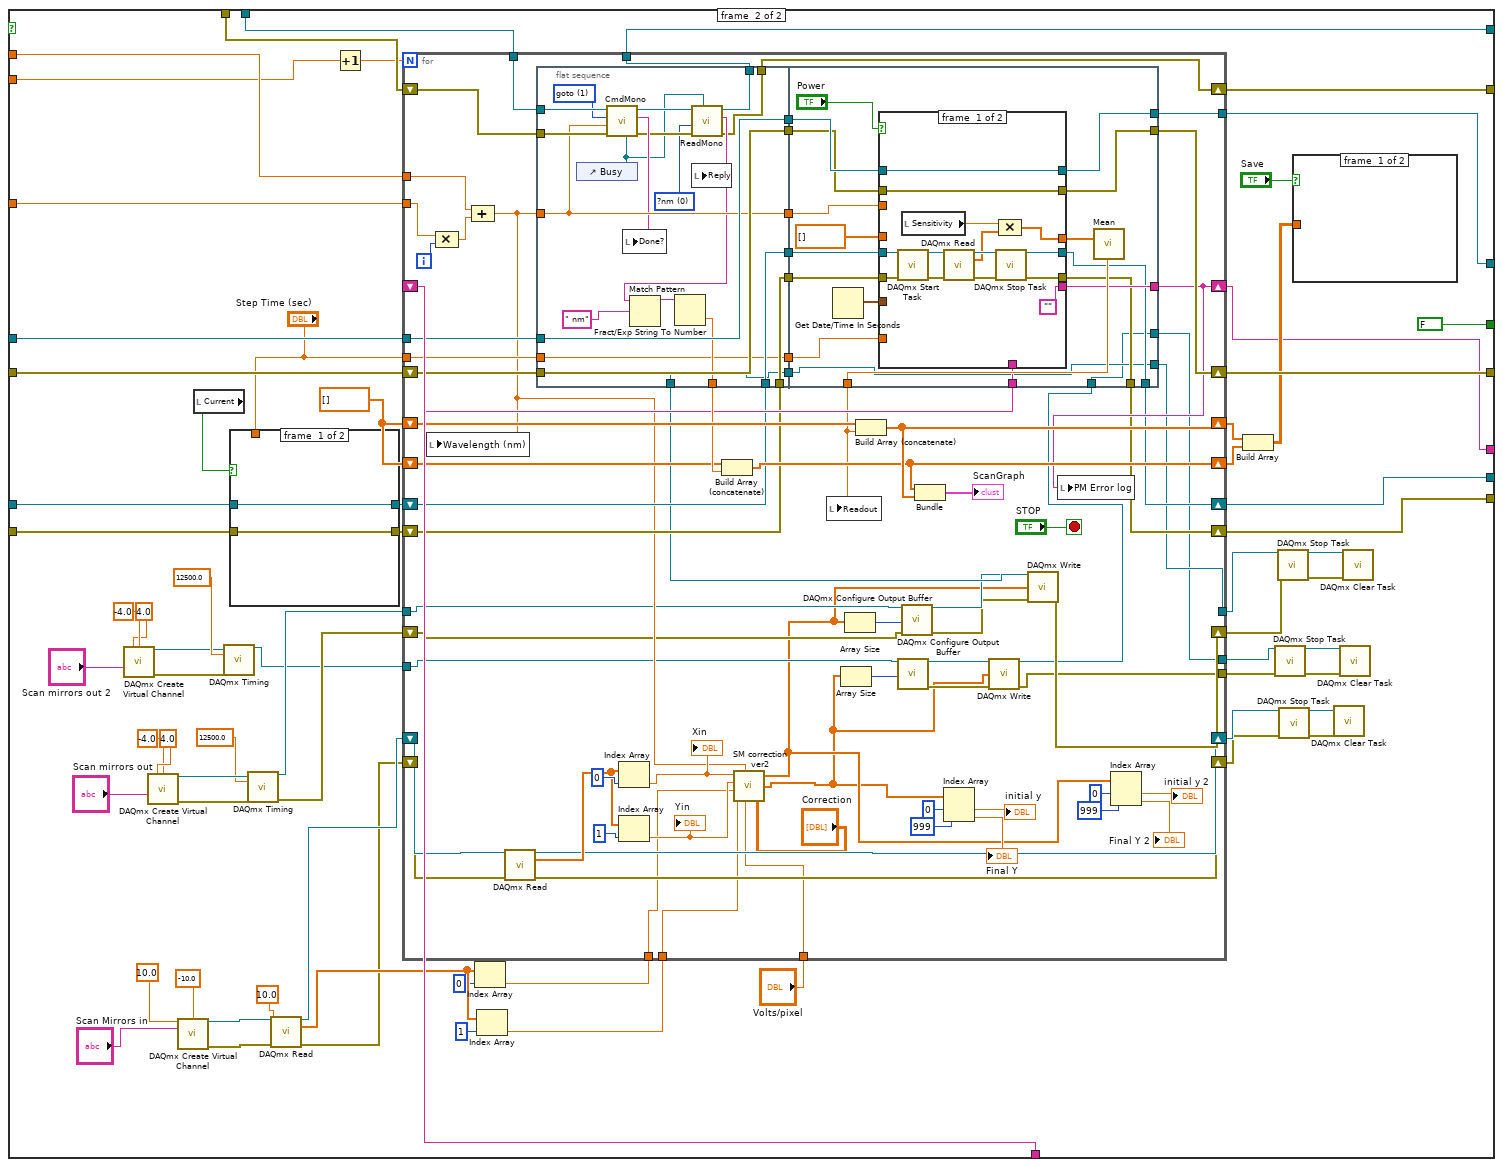
[diagram p15: hidden frame]
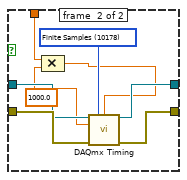
[diagram p16: hidden frame]
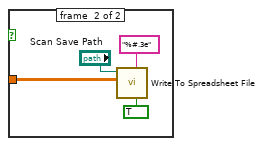
[diagram p17: hidden frame]
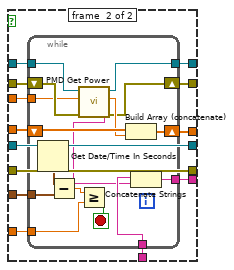
[diagram p18: hidden frame]
diagram:
  n1 = flat-sequence {
    tunnel: [w39] -> w20
    tunnel: [w38] -> w19
    tunnel: [w37] -> w18
    tunnel: [w36] -> w17
    tunnel: [w23] -> w12
    tunnel: [w24] -> w9
    tunnel: [w29] -> w8
    tunnel: [w30] -> w7
    tunnel: [w28] -> w6
    tunnel: [w27] -> w5
    tunnel: w20 -> [w64]
    tunnel: w19 -> [w65]
    tunnel: w18 -> [w63]
    tunnel: w17 -> [w62]
    tunnel: [w61] -> w16
    tunnel: [w60] -> w15
    tunnel: [w59] -> w14
    tunnel: [w58] -> w13
    tunnel: w12 -> [w55]
    tunnel: [w46] -> w11
    tunnel: [w45] -> w10
    tunnel: w9 -> [w56]
    tunnel: w8 -> [w54]
    tunnel: w7 -> [w53]
    tunnel: w6 -> [w52]
    tunnel: w5 -> [w51]
    tunnel: [w47] -> w4
    tunnel: [w48] -> w3
    tunnel: [w49] -> w2
    tunnel: [w50] -> w1
    tunnel: w16 -> [w520]
    tunnel: w15 -> [w519]
    tunnel: w14 -> [w518]
    tunnel: w13 -> [w517]
    tunnel: w11 -> [w515]
    tunnel: w10 -> [w516]
    tunnel: w4 -> [w514]
    tunnel: w3 -> [w513]
    tunnel: w2 -> [w512]
    tunnel: w1 -> [w511]
    frame #0 {
      w25 = -10.0 ("minimum value")
      w26 = 10.0 ("maximum value")
      n2 = call "PM100D_Initialize.vi"() -> ("error out"=w43:errorcluster, "Instrument"=→"IDN String":string, "VISA out"=w44:refnum<visa-resource-name>)  [unwired: 2 in, 1 out]
      n3 = call-poly <vilib>:"DAQmx Create Virtual Channel.vi"("maximum value"=w26, "minimum value"=w25, "physical channels"="Output A") -> ("task out"=w30:refnum<k21>, "error out"=w29:errorcluster)  [unwired: 11 in]
      n4 = call-poly <vilib>:"DAQmx Create Virtual Channel.vi"("maximum value"=10.0, "minimum value"=-10.0, "physical channels"="Input Channel") -> ("task out"=w24:refnum<k21>, "error out"=w23:errorcluster)  [unwired: 11 in]
      n5 = call "PM100D_SensorFlag.vi"("error in (no error)"=w43, "VISA in"=w44) -> ("error out"=w39:errorcluster, "VISA out"=w38:refnum<visa-resource-name>, "sn"=→"Sensor SN":string, "name"=→"Sensor Name":string)  [unwired: 2 in, 4 out]
      n6 = call-poly <vilib>:"DAQmx Create Virtual Channel.vi"("maximum value"=w26, "minimum value"=w25, "physical channels"="Output B") -> ("task out"=w27:refnum<k21>, "error out"=w28:errorcluster)  [unwired: 11 in]
      n7 = call "OpenMono.vi"("Mono Port"="Mono Port") -> ("VISA resource name out"=w37:refnum<visa-resource-name>, "error out"=w36:errorcluster)
      "Busy" <- FALSE ("Busy")
    }
    frame #1 {
      n8 = while {
        tunnel: w65 -> [w86]
        tunnel: w63 -> [w88]
        tunnel: [w83] -> w60
        tunnel: [w81] -> w58
        shift-right: [w80] -> w59
        shift-left: w64 -> [w85]
        shift-right: [w82] -> w61
        shift-left: w62 -> [w87]
        shift-right: [w78] -> _
        shift-left: "" -> [w79]
        shift-right: [w67] -> w45
        shift-left: w55 -> [w76]
        shift-right: [w66] -> w46
        shift-left: w56 -> [w77]
        shift-right: [w68] -> w50
        shift-left: w53 -> [w75]
        shift-right: [w69] -> w49
        shift-left: w54 -> [w74]
        shift-right: [w70] -> w48
        shift-left: w51 -> [w72]
        shift-right: [w71] -> w47
        shift-left: w52 -> [w73]
        stop <- "Exit" stop-if-true
        n9 = stacked-sequence {
          seq-local: [w107 _ _] -> [_ w203 _]
          seq-local: [w112 _ _] -> [_ _ w256]
          seq-local: [w111 _ _] -> [_ _ w255]
          seq-local: [_ w210 _] -> [_ _ w254]
          seq-local: [_ w211 _] -> [_ _ w253]
          seq-local: [_ w204 _] -> [_ _ w247]
          seq-local: [_ w198 _] -> [_ _ w243]
          seq-local: [_ w199 _] -> [_ _ w242]
          tunnel: w88 -> [w118 _ _]
          tunnel: w87 -> [w117 _ _]
          tunnel: w86 -> [_ w213 _]
          tunnel: w85 -> [_ w212 _]
          tunnel: [_ _ w252] -> w83
          tunnel: [_ _ w251] -> w82
          tunnel: [_ _ w250] -> w81
          tunnel: [_ _ w249] -> w80
          tunnel: w79 -> [_ w206 _]
          tunnel: [_ _ w246] -> w78
          tunnel: w77 -> [_ w197 _]
          tunnel: w76 -> [_ w196 _]
          tunnel: [_ _ w245] -> w66
          tunnel: [_ _ w244] -> w67
          tunnel: w75 -> [w102 _ _]
          tunnel: w74 -> [w103 _ _]
          tunnel: w73 -> [w105 _ _]
          tunnel: w72 -> [w104 _ _]
          tunnel: [w101 _ _] -> w71
          tunnel: [w100 _ _] -> w70
          tunnel: [w99 _ _] -> w69
          tunnel: [w98 _ _] -> w68
          frame #0 {
            # "Wavelength"
            n10 = while {
              shift-right: [w140] -> w89
              shift-left: _ -> [w139]
              tunnel: "Voltage B" -> [w140]
              tunnel: [w139] -> w94
              tunnel: "Voltage A" -> [w138]
              shift-right: [w138] -> w90
              shift-left: _ -> [w137]
              tunnel: [w137] -> w95
              stop <- TRUE stop-if-true
            }
            n11 = case shown="False" "Send Question" {
              tunnel: w118 -> [w188 w194]
              tunnel: w117 -> [w187 w193]
              tunnel: [w188 w192] -> w120
              tunnel: [w187 w191] -> w119
              frame #0 {
                (unwired) FALSE ("Read Error")
              }
              frame #1 {
                n12 = control-ref of="Busy"() -> (w189:refnum<vi>)
                n13 = call "ReadMono.vi"("Busy"=w189, "error in (no error)"=w193, "Cmd"="Ask?", "Mono Port"=w194) -> ("error out"=w191:errorcluster, "Response"=→"Reply":string, "Mono Port Out"=w192:refnum<visa-resource-name>)  [unwired: 2 in, 1 out]
              }
            }
            n14 = Not Equal?(x=w90, y=w95) -> (x != y?=w93:bool)
            n15 = Not Equal?(x=w89, y=w94) -> (x != y?=w92:bool)
            n16 = Or(x=w93, y=w92) -> (x .or. y?=w91:bool)
            n17 = case shown="False" w91 {
              tunnel: w105 -> [w123 w136]
              tunnel: w104 -> [w124 w135]
              tunnel: w103 -> [w125 w134]
              tunnel: w102 -> [w126 w133]
              tunnel: [w123 w132] -> w101
              tunnel: [w124 w131] -> w100
              tunnel: [w125 w130] -> w99
              tunnel: [w126 w129] -> w98
              tunnel: w90 -> [_ w127]
              tunnel: w89 -> [_ w128]
              frame #0 {
              }
              frame #1 {
                n18 = call-poly <vilib>:"DAQmx Write.vi"("task/channels in"=w135, "data"=w128, "error in"=w136) -> ("task out"=w131:refnum<k21>, "error out"=w132:errorcluster)  [unwired: 10 in, 1 out]
                n19 = call-poly <vilib>:"DAQmx Write.vi"("task/channels in"=w133, "data"=w127, "error in"=w134) -> ("task out"=w129:refnum<k21>, "error out"=w130:errorcluster)  [unwired: 10 in, 1 out]
              }
            }
            n20 = case shown="False" "Send Command" {
              tunnel: w120 -> [w173 w186]
              tunnel: w119 -> [w172 w185]
              tunnel: [w173 w178] -> w115
              tunnel: [w172 w177] -> w114
              tunnel: "Wavelength (nm)" -> [w171 w181]
              tunnel: [w171 w181] -> w113
              frame #0 {
              }
              frame #1 {
                w176 = u16 0 items=["?nm", "?nm/min", "?grating", "?turret", "?gratings"] ("Cmd")
                n21 = control-ref of="Busy"() -> (w174:refnum<vi>)
                n22 = call "CmdMono.vi"("Busy"=w174, "Scan Speed (nm/min)"="Scan Speed (nm/min)", "error in (no error)"=w185, "Wavelength (nm)"=w181, "Cmd"="Command", "Mono Port"=w186) -> ("error out"=w179:errorcluster, "Response"=→"Done?":string, "Mono Port Out"=w180:refnum<visa-resource-name>)  [unwired: 2 in, 1 out]
                n23 = call "ReadMono.vi"("Busy"=w174, "error in (no error)"=w179, "Cmd"=w176, "Mono Port"=w180) -> ("error out"=w177:errorcluster, "Response"=w175:string, "Mono Port Out"=w178:refnum<visa-resource-name>)  [unwired: 2 in, 1 out]
                n24 = local write "Reply"(w175) -> ()
              }
            }
            n25 = case shown="False" "Step" {
              tunnel: w115 -> [w151 w170]
              tunnel: w114 -> [w150 w169]
              tunnel: w113 -> [w149 w163]
              tunnel: [w151 w156] -> w112
              tunnel: [w150 w157] -> w111
              tunnel: "Increment (nm)" -> [_ w162]
              tunnel: [w149 w152] -> w107
              frame #0 {
              }
              frame #1 {
                w154 = u16 0 items=["?nm", "?nm/min", "?grating", "?turret", "?gratings"] ("Cmd")
                w161 = u16 1 items=["nm", "goto", "nm/min", "VIS grating", "IR grating"] ("Cmd")
                n26 = Select(t=1, s="Up", f=-1) -> (s? t:f=w168:i32)
                n27 = control-ref of="Busy"() -> (w153:refnum<vi>)
                n28 = Compound Arithmetic op=MULTIPLY(w168, w162) -> (w164:dbl)
                n29 = Compound Arithmetic op=ADD(w164, w163) -> (w152:dbl)
                n30 = call "CmdMono.vi"("Busy"=w153, "error in (no error)"=w169, "Wavelength (nm)"=w152, "Cmd"=w161, "Mono Port"=w170) -> ("error out"=w158:errorcluster, "Response"=w160:string, "Mono Port Out"=w159:refnum<visa-resource-name>)  [unwired: 3 in, 1 out]
                n31 = call "ReadMono.vi"("Busy"=w153, "error in (no error)"=w158, "Cmd"=w154, "Mono Port"=w159) -> ("error out"=w157:errorcluster, "Response"=w155:string, "Mono Port Out"=w156:refnum<visa-resource-name>)  [unwired: 2 in, 1 out]
                n32 = local write "Done?"(w160) -> ()
                n33 = local write "Reply"(w155) -> ()
              }
            }
            n34 = event shown="[0] Timeout" {
              selector: _ -> [_ _]
              dyn-events: _ -> [_ _]
              timeout: 0 -> [_ _]
              event #0 {
                n35 = event-data() -> ()  [unwired: 1 in, 2 out]
              }
              event #1 {
                n36 = event-data() -> ()  [unwired: 1 in, 1 out]
                n37 = local write "Done?"("   ..." ("Done?")) -> ()
              }
            }
            n38 = event shown="[0] Timeout" {
              selector: _ -> [_ _ _]
              dyn-events: _ -> [_ _ _]
              timeout: 0 -> [_ _ _]
              event #0 {
                n39 = event-data() -> ()  [unwired: 1 in, 2 out]
              }
              event #1 {
                n40 = event-data() -> ()  [unwired: 1 in, 7 out]
                n41 = local read "Power"() -> (w142:bool)
                n42 = case shown="False" w142 {
                  selector: w142 -> [w144 _]
                  frame #0 {
                    w143 = "Power (W)" ("Y Scale.Name Label.Text")
                    n43 = local write "Current"(w144) -> ()
                    n44 = property on="ScanGraph" class="XYGraph (strict)"("YScale.NameLbl.Text"=w143) -> ()  [unwired: 2 in, 2 out]
                    n45 = property on="Waveform Chart" class="WFChart (strict)"("YScale.NameLbl.Text"=w143) -> ()  [unwired: 2 in, 2 out]
                  }
                  frame #1 {
                  }
                }
                n46 = event-data("Discard?"=w142) -> ()  [unwired: 1 in, 1 out]
              }
              event #2 {
                n47 = event-data() -> ()  [unwired: 1 in, 7 out]
                n48 = local read "Current"() -> (w145:bool)
                n49 = case shown="False" w145 {
                  selector: w145 -> [w146 _]
                  frame #0 {
                    w147 = "Current (A)" ("Y Scale.Name Label.Text")
                    n50 = local write "Power"(w146) -> ()
                    n51 = property on="ScanGraph" class="XYGraph (strict)"("YScale.NameLbl.Text"=w147) -> ()  [unwired: 2 in, 2 out]
                    n52 = property on="Waveform Chart" class="WFChart (strict)"("YScale.NameLbl.Text"=w147) -> ()  [unwired: 2 in, 2 out]
                  }
                  frame #1 {
                  }
                }
                n53 = event-data("Discard?"=w145) -> ()  [unwired: 1 in, 1 out]
              }
            }
          }
          frame #1 {
            # "Wavelength"
            n54 = control-ref of="Zero?"() -> (w208:refnum<vi>)
            n55 = call "PMD Settings.vi"("Visa In"=w213, "Zero?"=w208, "PMD Settings In"="PMD Settings", "Error In"=w212, "Range"="Range") -> ("AUTO?"=→"AUTO?":bool, "Rng"=→"Rng":string, "Visa Out"=w216:refnum<visa-resource-name>, "ZeroValue"=→"Zero Value":dbl, "PM Error log"=w207:string, "error out"=w215:errorcluster)
            n56 = local write "Wavelength (nm)"(w203) -> ()
            n57 = call "PMD Get Power.vi"("VISA In"=w216, "Wavelength (nm)"=w203, "error in"=w215) -> ("PMD Error"=w205:string, "VISA out"=w210:refnum<visa-resource-name>, "Readout value"=w202:dbl, "error out"=w211:errorcluster)  [unwired: 1 in, 2 out]
            n58 = case shown="False" "Current" {
              tunnel: w202 -> [w223 _]
              tunnel: w197 -> [w222 w226]
              tunnel: w196 -> [w221 w227]
              tunnel: [w223 w239] -> w200
              tunnel: [w221 w235] -> w198
              tunnel: [w222 w236] -> w199
              frame #0 {
              }
              frame #1 {
                w229 = 10178 items=["Finite Samples"=10178, "Continuous Samples"=10123, "Hardware Timed Single Point"=12522] ("sample mode")
                n59 = call-poly <vilib>:"DAQmx Timing.vi"("task/channels in"=w226, "sample mode"=w229, "samples per channel"=50, "rate"=1000.0, "error in"=w227) -> ("task out"=w225:refnum<k21>, "error out"=w224:errorcluster)  [unwired: 9 in]
                n60 = call <vilib>:"DAQmx Start Task.vi"("task/channels in"=w225, "error in"=w224) -> ("task out"=w237:refnum<k21>, "error out"=w238:errorcluster)  [unwired: 12 in]
                n61 = call-poly <vilib>:"DAQmx Read.vi"("task/channels in"=w237, "error in"=w238) -> ("task out"=w233:refnum<k21>, "data"=w232:dbl[], "error out"=w234:errorcluster)  [unwired: 11 in]
                n62 = call <vilib>:"Mean.vi"("X"=w232) -> ("mean"=w231:dbl)  [unwired: 1 out]
                n63 = Compound Arithmetic op=MULTIPLY("Sensitivity", w231) -> (w239:dbl)
                n64 = call <vilib>:"DAQmx Stop Task.vi"("task/channels in"=w233, "error in"=w234) -> ("task out"=w236:refnum<k21>, "error out"=w235:errorcluster)  [unwired: 12 in]
              }
            }
            "Readout" <- w200
            n65 = Concatenate Strings(w206, w207, w205) -> (w204:string)
            n66 = case shown="False" "On" {
              tunnel: w200 -> [_ w241]
              frame #0 {
              }
              frame #1 {
                "Waveform Chart" <- w241
              }
            }
          }
          frame #2 {
            # "Wavelength"
            n67 = Subtract(x="End", y="Start") -> (x-y=w261:dbl)
            n68 = Divide(x=w261, y="Step Size (nm)") -> (x/y=w260:dbl)
            n69 = Round To Nearest(number=w260) -> (nearest integer value=w259:dbl)
            n70 = case shown="True" "Scan" {
              tunnel: w259 -> [_ w335]
              tunnel: w255 -> [w269 w337]
              tunnel: w256 -> [w268 w338]
              tunnel: "Start" -> [_ w340]
              tunnel: "Step Size (nm)" -> [_ w339]
              tunnel: w254 -> [w271 w333]
              tunnel: w253 -> [w270 w332]
              tunnel: [w271 w321] -> w250
              tunnel: [w270 w331] -> w249
              tunnel: [w269 w330] -> w251
              tunnel: [w268 w329] -> w252
              tunnel: [FALSE ("Scan") FALSE ("Scan")] -> w248
              tunnel: w247 -> [w266 w323]
              tunnel: [w266 w322] -> w246
              tunnel: [w265 w320] -> w245
              tunnel: [w264 w319] -> w244
              tunnel: w243 -> [w264 w317]
              tunnel: w242 -> [w265 w316]
              frame #0 {
              }
              frame #1 {
                w336 = dbl[] []
                n71 = call-poly <vilib>:"DAQmx Create Virtual Channel.vi"("maximum value"=4.0, "minimum value"=-4.0, "physical channels"="Scan mirrors out 2") -> ("task out"=w282:refnum<k21>, "error out"=w283:errorcluster)  [unwired: 11 in]
                n72 = call-poly <vilib>:"DAQmx Create Virtual Channel.vi"("maximum value"=4.0, "minimum value"=-4.0, "physical channels"="Scan mirrors out") -> ("task out"=w296:refnum<k21>, "error out"=w294:errorcluster)  [unwired: 11 in]
                n73 = call-poly <vilib>:"DAQmx Create Virtual Channel.vi"("maximum value"=10.0, "minimum value"=-10.0, "physical channels"="Scan Mirrors in") -> ("task out"=w307:refnum<k21>, "error out"=w311:errorcluster)  [unwired: 11 in]
                n74 = local read "Current"() -> (w318:bool)
                n75 = call-poly <vilib>:"DAQmx Timing.vi"("task/channels in"=w282, "rate"=12500.0, "error in"=w283) -> ("task out"=w278:refnum<k21>)  [unwired: 11 in, 1 out]
                n76 = case shown="False" w318 {
                  tunnel: w317 -> [w341 w349]
                  tunnel: w316 -> [w342 w348]
                  tunnel: [w342 w347] -> w315
                  tunnel: [w341 w346] -> w314
                  tunnel: "Step Time (sec)" -> [_ w345]
                  frame #0 {
                  }
                  frame #1 {
                    w350 = 10178 items=["Finite Samples"=10178, "Continuous Samples"=10123, "Hardware Timed Single Point"=12522] ("sample mode")
                    w344 = 1000.0 ("rate")
                    n77 = Compound Arithmetic op=MULTIPLY(w345, w344) -> (w343:dbl)
                    n78 = call-poly <vilib>:"DAQmx Timing.vi"("task/channels in"=w348, "sample mode"=w350, "samples per channel"=w343, "rate"=w344, "error in"=w349) -> ("task out"=w347:refnum<k21>, "error out"=w346:errorcluster)  [unwired: 9 in]
                  }
                }
                n79 = call-poly <vilib>:"DAQmx Timing.vi"("task/channels in"=w296, "rate"=12500.0, "error in"=w294) -> ("task out"=w295:refnum<k21>, "error out"=w293:errorcluster)  [unwired: 11 in]
                n80 = call-poly <vilib>:"DAQmx Read.vi"("task/channels in"=w307, "timeout"=10.0, "error in"=w311) -> ("task out"=w292:refnum<k21>, "data"=w306:dbl[], "error out"=w291:errorcluster)  [unwired: 10 in]
                n81 = Increment(x=w335) -> (x+1=w334:dbl)
                n82 = Index Array(array=w306, index=0) -> (element=w303:dbl)
                n83 = Index Array(array=w306, index=1) -> (element=w302:dbl)
                n84 = for {
                  N: w334 -> [_]
                  tunnel: w338 -> [w425]
                  tunnel: w340 -> [w421]
                  tunnel: w339 -> [w423]
                  shift-right: [w409] -> w328
                  shift-left: w336 -> [w427]
                  shift-right: [w420] -> w330
                  shift-left: w337 -> [w426]
                  shift-right: [w406] -> w327
                  shift-left: w336 -> [w407]
                  tunnel: w333 -> [w418]
                  shift-right: [w413] -> w331
                  shift-left: w332 -> [w417]
                  tunnel: [w412] -> w321
                  tunnel: [w411] -> w329
                  shift-right: [w404] -> w322
                  shift-left: w323 -> [w405]
                  shift-right: [w401] -> w319
                  shift-left: w314 -> [w396]
                  shift-right: [w400] -> w320
                  shift-left: w315 -> [w397]
                  tunnel: "Step Time (sec)" -> [w398]
                  tunnel: w303 -> [w384]
                  tunnel: w302 -> [w383]
                  shift-right: [w391] -> w297
                  shift-left: w293 -> [w373]
                  shift-right: [w390] -> w290
                  shift-left: w292 -> [w389]
                  shift-right: [w387] -> w289
                  shift-left: w291 -> [w388]
                  tunnel: "Volts/pixel" -> [w377]
                  tunnel: w295 -> [w375]
                  tunnel: [w380] -> w298
                  tunnel: w278 -> [w360]
                  tunnel: [w358] -> w273
                  tunnel: [w357] -> w272
                  i -> [w424]
                  stop <- "STOP" stop-if-true
                  n85 = Compound Arithmetic op=MULTIPLY(w423, w424) -> (w422:dbl)
                  n86 = Compound Arithmetic op=ADD(w421, w422) -> (w382:dbl)
                  n87 = local write "Wavelength (nm)"(w382) -> ()
                  n88 = call-poly <vilib>:"DAQmx Read.vi"("task/channels in"=w389, "error in"=w388) -> ("task out"=w390:refnum<k21>, "data"=w392:dbl[], "error out"=w387:errorcluster)  [unwired: 11 in]
                  n89 = flat-sequence {
                    tunnel: w426 -> [w448]
                    tunnel: w425 -> [w447]
                    tunnel: w382 -> [w443]
                    tunnel: [w432] -> w420
                    tunnel: w418 -> [w445]
                    tunnel: w417 -> [w444]
                    tunnel: [w445] -> w416
                    tunnel: [w444] -> w415
                    tunnel: [w443] -> w414
                    tunnel: [w437] -> w411
                    tunnel: [w433] -> w408
                    tunnel: w396 -> [w430]
                    tunnel: [w431] -> w403
                    tunnel: w397 -> [w431]
                    tunnel: [w430] -> w402
                    tunnel: [w429] -> w399
                    tunnel: w398 -> [w429]
                    tunnel: w379 -> [w428]
                    tunnel: [w428] -> w378
                    tunnel: [w464] -> w395
                    tunnel: w416 -> [w463]
                    tunnel: w415 -> [w462]
                    tunnel: w414 -> [w461]
                    tunnel: [w457] -> w413
                    tunnel: [w460] -> w412
                    tunnel: w405 -> [w459]
                    tunnel: [w458] -> w404
                    tunnel: w403 -> [w455]
                    tunnel: w402 -> [w454]
                    tunnel: [w452] -> w400
                    tunnel: [w453] -> w401
                    tunnel: w399 -> [w456]
                    tunnel: [w450] -> w380
                    tunnel: w378 -> [w450]
                    tunnel: [w449] -> w358
                    tunnel: w359 -> [w449]
                    frame #0 {
                      w439 = u16 0 items=["?nm", "?nm/min", "?grating", "?turret", "?gratings"] ("Cmd")
                      w446 = u16 1 items=["nm", "goto", "nm/min", "VIS grating", "IR grating"] ("Cmd")
                      n90 = control-ref of="Busy"() -> (w438:refnum<vi>)
                      n91 = call "CmdMono.vi"("Busy"=w438, "error in (no error)"=w448, "Wavelength (nm)"=w443, "Cmd"=w446, "Mono Port"=w447) -> ("error out"=w440:errorcluster, "Response"=w442:string, "Mono Port Out"=w441:refnum<visa-resource-name>)  [unwired: 3 in, 1 out]
                      n92 = local write "Done?"(w442) -> ()
                      n93 = call "ReadMono.vi"("Busy"=w438, "error in (no error)"=w440, "Cmd"=w439, "Mono Port"=w441) -> ("error out"=w432:errorcluster, "Response"=w435:string, "Mono Port Out"=w437:refnum<visa-resource-name>)  [unwired: 2 in, 1 out]
                      n94 = Match Pattern(string=w435, regular expression=" nm") -> (before substring=w434:string)  [unwired: 1 in, 3 out]
                      n95 = Fract/Exp String To Number(string=w434) -> (number=w433:dbl)  [unwired: 3 in, 1 out]
                      n96 = local write "Reply"(w435) -> ()
                    }
                    frame #1 {
                      n97 = Get Date/Time In Seconds() -> (seconds since 1Jan1904=w466:timestamp)
                      n98 = case shown="True" "Power" {
                        tunnel: dbl[] [] -> [_ w494]
                        tunnel: w466 -> [_ w493]
                        tunnel: [w468 w492] -> w465
                        tunnel: w463 -> [w480 w491]
                        tunnel: w462 -> [w479 w490]
                        tunnel: w461 -> [_ w489]
                        tunnel: [w480 w488] -> w460
                        tunnel: w459 -> [_ w487]
                        tunnel: ["" w486] -> w458
                        tunnel: [w479 w485] -> w457
                        tunnel: w456 -> [_ w484]
                        tunnel: w455 -> [w478 w482]
                        tunnel: w454 -> [w477 w483]
                        tunnel: [w472 w483] -> w453
                        tunnel: [w471 w482] -> w452
                        frame #0 {
                          n99 = call <vilib>:"DAQmx Start Task.vi"("task/channels in"=w478, "error in"=w477) -> ("task out"=w476:refnum<k21>, "error out"=w475:errorcluster)  [unwired: 12 in]
                          n100 = local read "Sensitivity"() -> (w469:dbl)
                          n101 = call-poly <vilib>:"DAQmx Read.vi"("task/channels in"=w476, "error in"=w475) -> ("task out"=w474:refnum<k21>, "data"=w470:dbl[], "error out"=w473:errorcluster)  [unwired: 11 in]
                          n102 = call <vilib>:"DAQmx Stop Task.vi"("task/channels in"=w474, "error in"=w473) -> ("task out"=w471:refnum<k21>, "error out"=w472:errorcluster)  [unwired: 12 in]
                          n103 = Compound Arithmetic op=MULTIPLY(w469, w470) -> (w468:dbl[])
                        }
                        frame #1 {
                          n104 = while {
                            shift-right: [w509] -> w492
                            shift-left: w494 -> [w510]
                            tunnel: w493 -> [w507]
                            tunnel: w491 -> [w502]
                            tunnel: w489 -> [w498]
                            tunnel: [w500] -> w488
                            tunnel: w487 -> [w504]
                            tunnel: [w503] -> w486
                            shift-right: [w496] -> w485
                            shift-left: w490 -> [w501]
                            tunnel: w484 -> [w495]
                            stop <- w505 stop-if-true
                            n105 = Get Date/Time In Seconds() -> (seconds since 1Jan1904=w508:timestamp)
                            n106 = Subtract(x=w508, y=w507) -> (x-y=w506:dbl)
                            n107 = call "PMD Get Power.vi"("VISA In"=w502, "Wavelength (nm)"=w498, "error in"=w501) -> ("PMD Error"=w497:string, "VISA out"=w500:refnum<visa-resource-name>, "Readout value"=w499:dbl, "error out"=w496:errorcluster)  [unwired: 1 in, 2 out]
                            n108 = Greater Or Equal?(x=w506, y=w495) -> (x >= y?=w505:bool)
                            n109 = Build Array (concatenate)(w510, w499) -> (w509:dbl[])
                            n110 = Concatenate Strings(w504, w497) -> (w503:string)
                          }
                        }
                      }
                      n111 = call <vilib>:"Mean.vi"("X"=w465) -> ("mean"=w464:dbl)  [unwired: 1 out]
                    }
                  }
                  n112 = Index Array(array=w392, index=0) -> (element=w386:dbl)
                  "Xin" <- w386
                  n113 = Index Array(array=w392, index=1) -> (element=w385:dbl)
                  "Yin" <- w385
                  n114 = Build Array (concatenate)(w407, w408) -> (w406:dbl[])
                  n115 = call "SM correction ver2.vi"("V in x"=w386, "nm in"=w382, "V in y"=w385, "V x initial"=w384, "Volts/pixel"=w377, "V y initial"=w383, "Array"="Correction") -> ("V out x"=w356:dbl[], "V out y"=w355:dbl[])
                  n116 = local write "Readout"(w395) -> ()
                  n117 = Array Size(array=w355) -> (size(s)=w361:i32)
                  n118 = Array Size(array=w356) -> (size(s)=w376:i32)
                  n119 = Build Array (concatenate)(w427, w395) -> (w409:dbl[])
                  n120 = call <vilib>:"DAQmx Configure Output Buffer.vi"("task/channels in"=w360, "buffer size (in samples per channel)"=w361) -> ("task out"=w362:refnum<k21>, "error out"=w363:errorcluster)  [unwired: 12 in]
                  n121 = call <vilib>:"DAQmx Configure Output Buffer.vi"("task/channels in"=w375, "buffer size (in samples per channel)"=w376, "error in"=w373) -> ("task out"=w374:refnum<k21>, "error out"=w372:errorcluster)  [unwired: 11 in]
                  n122 = Bundle(w406, w409) -> (→"ScanGraph":cluster{dbl[], dbl[]})  [unwired: 1 in]
                  n123 = Index Array(array=w355, index #1=0 ("index"), index #2=999 ("index")) -> (element #1=→"initial y":dbl, element #2=→"Final Y":dbl)
                  n124 = call-poly <vilib>:"DAQmx Write.vi"("task/channels in"=w362, "data"=w355, "error in"=w363) -> ("task out"=w359:refnum<k21>, "error out"=w357:errorcluster)  [unwired: 10 in, 1 out]
                  n125 = call-poly <vilib>:"DAQmx Write.vi"("task/channels in"=w374, "data"=w356, "error in"=w372) -> ("task out"=w379:refnum<k21>, "error out"=w391:errorcluster)  [unwired: 10 in, 1 out]
                  n126 = local write "PM Error log"(w404) -> ()
                  n127 = Index Array(array=w356, index #1=0 ("index"), index #2=999 ("index")) -> (element #1=→"initial y 2":dbl, element #2=→"Final Y 2":dbl)
                }
                n128 = Build Array(w328, w327) -> (w326:dbl[][])
                n129 = call <vilib>:"DAQmx Stop Task.vi"("task/channels in"=w273, "error in"=w272) -> ("task out"=w274:refnum<k21>, "error out"=w275:errorcluster)  [unwired: 12 in]
                n130 = call <vilib>:"DAQmx Stop Task.vi"("task/channels in"=w298, "error in"=w297) -> ("task out"=w286:refnum<k21>, "error out"=w285:errorcluster)  [unwired: 12 in]
                n131 = call <vilib>:"DAQmx Stop Task.vi"("task/channels in"=w290, "error in"=w289) -> ("task out"=w277:refnum<k21>, "error out"=w276:errorcluster)  [unwired: 12 in]
                n132 = case shown="False" "Save" {
                  tunnel: w326 -> [_ w351]
                  frame #0 {
                  }
                  frame #1 {
                    n133 = call-poly <vilib>:"Write To Spreadsheet File.vi"("transpose? (no:F)"=TRUE, "format (%.3f)"="%#.3e", "2D data"=w351, "file path (dialog if empty)"="Scan Save Path") -> ()  [unwired: 4 in, 1 out]
                  }
                }
                n134 = call <vilib>:"DAQmx Clear Task.vi"("task in"=w277, "error in"=w276) -> ()  [unwired: 13 in, 1 out]
                n135 = call <vilib>:"DAQmx Clear Task.vi"("task in"=w274, "error in"=w275) -> ()  [unwired: 13 in, 1 out]
                n136 = call <vilib>:"DAQmx Clear Task.vi"("task in"=w286, "error in"=w285) -> ()  [unwired: 13 in, 1 out]
              }
            }
            n137 = local write "Scan"(w248) -> ()
          }
        }
        "PM Error log" <- w78
      }
    }
    frame #2 {
      n138 = call <vilib>:"DAQmx Clear Task.vi"("task in"=w515, "error in"=w516) -> ()  [unwired: 13 in, 1 out]
      n139 = call <vilib>:"DAQmx Clear Task.vi"("task in"=w511, "error in"=w512) -> ()  [unwired: 13 in, 1 out]
      n140 = call <vilib>:"DAQmx Clear Task.vi"("task in"=w513, "error in"=w514) -> ()  [unwired: 13 in, 1 out]
      n141 = VISA Close(VISA resource name=w519, error in (no error)=w520) -> (error out=w521:errorcluster)
      n142 = call "PM100D_Close.vi"("error in (no error)"=w518, "VISA resource name"=w517) -> ()  [unwired: 2 in]
      n143 = call <vilib>:"Simple Error Handler.vi"("error in (no error)"=w521) -> ()  [unwired: 1 in, 8 out]
    }
  }
